vi "SerialPort.Manager.vi"(11 "Module Config":T4={"Name"="Serial Port", "Parent Q"=refnum, "Is Child?"=FALSE, "Index"=0, "Dirs"={"Root"=path "", "Config"=path "C:/ATE/Config", "Logs"=path "C:/ATE/Logs", "Reports"=path "C:/ATE/Reports", "App Data"=path "C:/ProgramData/MAIN"}, "Simulate"=FALSE, "SimCtrl"=refnum}) -> ()   [LabVIEW 2018]
uses:
  <vilib>/KATE/Module/Module Config.ctl
  <vilib>/KATE/Queues/Q.Element.ctl
  <vilib>/KATE/Module/Module.Working Dirs.ctl
  Controls/SerialPort.Status Enum.ctl
  Controls/SeroalPort.Config Settings.ctl
  <vilib>/KATE/Event Log/Event Notification/Event Log.Log Level.ctl
  <vilib>/KATE/Module/Module.SW Version Info.ctl
  <vilib>/KATE/Module/Window/Window.Task, Action.ctl
  Class/SerialPort.lvclass
  Controls/SerialPort.Parent Task Names.ctl
  Utils/Functions/FunctMgr/FunctMgr.lvclass
  <vilib>/Utility/sysdir.llb/System Directory Type.ctl
  <vilib>/KATE/Event Log/Event Notification/Event Log.Notification Type.ctl
  <vilib>/Utility/config.llb/Read Key (String).vi
  <vilib>/KATE/Config/Stored Controls/Class.SaveCtrls.lvclass
  <vilib>/KATE/Queues/Queue Utils.lvlib
  <vilib>/KATE/Module/Module Utils.lvlib
  <vilib>/KATE/Event Log/Event Log.lvlib
  <vilib>/KATE/Scheduler/Scheduler.lvlib
  <vilib>/KATE/Menu/Menu Utils.lvlib
  <vilib>/KATE/Config/Config Utils.lvlib
  <vilib>/KATE/Status/Status Utils.lvlib
  <vilib>/KATE/Files/File Utils.lvlib
  <vilib>/KATE/SeqMgr/SeqMgr.lvlib
  <vilib>/KATE/Event Log/Event Notification/Event Notification.lvclass
  <vilib>/Utility/config.llb/NI_LVConfig.lvlib
panel:
  in  "Main Tab":enum32{"Operate", "Maint"}(tab)
  in  "Data Tab":enum32{"Read/Write", "Config"}(tab)
  in  "Send Tab":bool
  in  "Save Log":bool
  out "Error Status":string
  in  "Clear Log":bool
  in  "Write":string
  out "Log":string
  in  "Log Size (Chars)":i32=100000
  in  "Auto Scroll":bool=TRUE
  out "Simulate Indication":string="Simulating Instruments"
  out "Q Dur ms":u32=100 caption="Dur(ms)"
  in  "Q Timeout ms":u32=5000 caption="Timeout ms"
  in  "Query":bool
  out "Q Data":string
  in  "Q Cmd":string="id" caption="Cmd"
  in  "Q MsgEnd":string="lhtx>" caption="MsgEnd"
  in  "VID":string="28DE"
  in  "PID":string
  in  "TermChar":string="\n\r" caption="Command Term Char"
  in  "Timeout ms (3sec)":u32=3000
  in  "Config":T1={"Baud Rate (115200)"=115200, "Data Bits (8)"=8, "Parity (0:none)"=enum."None", "Stop Bits (10: 1 bit)"=10, "Flow Control (0:none)"=enum."None", "Enable Term Char (T)"=TRUE, "Term Char(0xA = '\\n' = LF) "=10} {"Term Char(0xA = '\\n' = LF)" format="%.0x"; "Stop Bits (10: 1 bit)" items=["1.0"=10, "1.5"=15, "2.0"=20]; "Data Bits (8)" min=5 max=8 step=1}
  out "Status":string
  out "Error":errorcluster
  in  "Auto Find Port":bool=TRUE caption="Auto"
  in  "Logging Level":T2
  out "Rev":string="v1.0.0"
  in  "COM Port":refnum<visa-resource-name>
  in  "Disconnect":bool
  in  "Connect":bool
  out "State":T3
  in  "Leave Maint":bool
  # "Serial Port Manager"
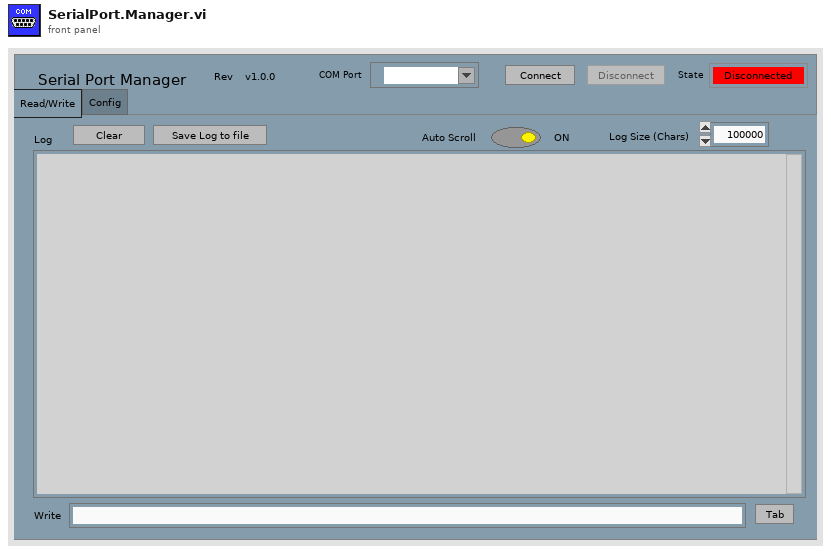
[diagram p1: front panel]
types:
  T1 = typedef "SeroalPort.Config Settings.ctl" = cluster{"Baud Rate (115200)":u32, "Data Bits (8)":u16, "Parity (0:none)":enum16{"None", "Odd", "Even", "Mark", "Space"}, "Stop Bits (10: 1 bit)":u16, "Flow Control (0:none)":enum16{"None", "XON/XOFF", "RTS/CTS", "XON/XOFF & RTS/CTS", "DTR/DSR", "XON/XOFF & DTR/DSR"}, "Enable Term Char (T)":bool, "Term Char(0xA = '\\n' = LF) ":u8}
  T2 = typedef "KATE_Lib.lvlib/Event Log.lvlib/Event Log.Log Level.ctl" = enum16{"Normal", "Verbose", "Debug0", "Debug1", "Debug2"}
  T3 = typedef "SerialPort.Status Enum.ctl" = enum16{"Disconnected", "Connecting", "Connected"}
  T4 = typedef "KATE_Lib.lvlib/Module Utils.lvlib/Module Config.ctl" = cluster{"Name":string, "Parent Q":refnum<queue>, "Is Child?":bool, "Index":i32, "Dirs":T5, "Simulate":bool, "SimCtrl":refnum<vi>}
  T5 = typedef "KATE_Lib.lvlib/Module Utils.lvlib/Module.Working Dirs.ctl" = cluster{"Root":path, "Config":path, "Logs":path, "Reports":path, "App Data":path}
  T6 = typedef "KATE_Lib.lvlib/Module Utils.lvlib/Module.SW Version Info.ctl" = cluster{"AppName":string, "Company":string, "Version":string, "Description":string, "PN":string}
  T7 = typedef "KATE_Lib.lvlib/Module Utils.lvlib/Module Sys Info.ctl" = cluster{"Main Q":refnum<queue>, "Exe":bool, "SW Rev":T6, "Self Ref":refnum<vi>, "Main Tab":refnum<vi>, "Pane":refnum<vi>, "Stop":cluster{"Ref":refnum<event-registration>, "Event":refnum<user-event>}, "Cfg":T4, "Services":cluster{"Name":string, "vi ref":refnum<vi>}[], "Menu Ref":refnum<k9>, "CtrlStates":refnum<class "Class.SaveCtrls.lvclass">, "Docs":cluster{"Tags":string[], "Paths":path[]}, "Log":refnum<class "Event Notification.lvclass">, "Test Controls":refnum<vi>[], "Child Modules":cluster{"Name":string, "vi ref":refnum<vi>}[], "SW Items":string[][], "AppData":refnum<class "Class.AppData.lvclass">, "Subscriptions":refnum<class "Subscription.lvclass">}
  T8 = typedef "SerialPort.Parent Task Names.ctl" = cluster{"Rcv":string, "Event":string}
  T9 = enum8{"Enabled", "Disabled", "Disabled and Grayed Out"}
  T10 = enum16{"open", "replace", "create", "open or create", "replace or create", "replace or create with confirmation"}
  T11 = cluster{"Port Name":string, "Config":T1, "Port Timeout ms (3000)":u32}
  T12 = typedef "KATE_Lib.lvlib/Event Log.lvlib/Event Log.Notification Type.ctl" = enum16{"Normal", "Warning", "Error", "Success"}
  T13 = cluster{"Child Modules":cluster{"VI Ref":refnum<vi>, "Name":string}[]}
  T14 = cluster{"Local Error":errorcluster, "Lnch":bool, "TBD":string, "App":cluster{"Child Modules":cluster{"VI Ref":refnum<vi>, "Name":string}[]}, "SerialPort":refnum<class "SerialPort.lvclass">, "Log":string, "Parent Tasks":T8, "FunctMgr":refnum<class "FunctMgr.lvclass">, "Ctrl Lock":bool}
  T15 = typedef "NI_LVConfig.lvlib/Config Data RefNum.ctl" = refnum<k1>
  T16 = typedef "System Directory Type.ctl" = i32
  T17 = typedef "KATE_Lib.lvlib/Module Utils.lvlib/Window.Task, Action.ctl" = enum16{"Resize()", "Show Panel(Bool)", "Show Scroll Bars(Bool)", "Dock to SubPanel(SubPanel Ref)", "Undock from SubPanel()", "Return to SubPanel()", "Go To Maint Tab()", "Show Maint Tab(Bool)", "Open Block Diagram()"}
  T18 = typedef "eventvkey.ctl" = enum16{"ASCII", "Enter", "Return", "Shift", "Ctrl", "Alt", "Cmd", "Opt", "Caps", "NumLock", "Clear", "Break", "Up", "Down", "Left", "Right", "Insert", "Delete", "Home", "End", "PageUp", "PageDown", "Escape", "Help", "Pause", "ScrollLock", "F1", "F2", "F3", "F4", "F5", "F6", "F7", "F8", "F9", "F10", "F11", "F12", "F13", "F14", "F15", "F16", "F17", "F18", "F19", "F20", "F21", "F22", "F23", "F24", "Play", "VolumeUp", "VolumeDown", "Mute", "Two Byte Char"}
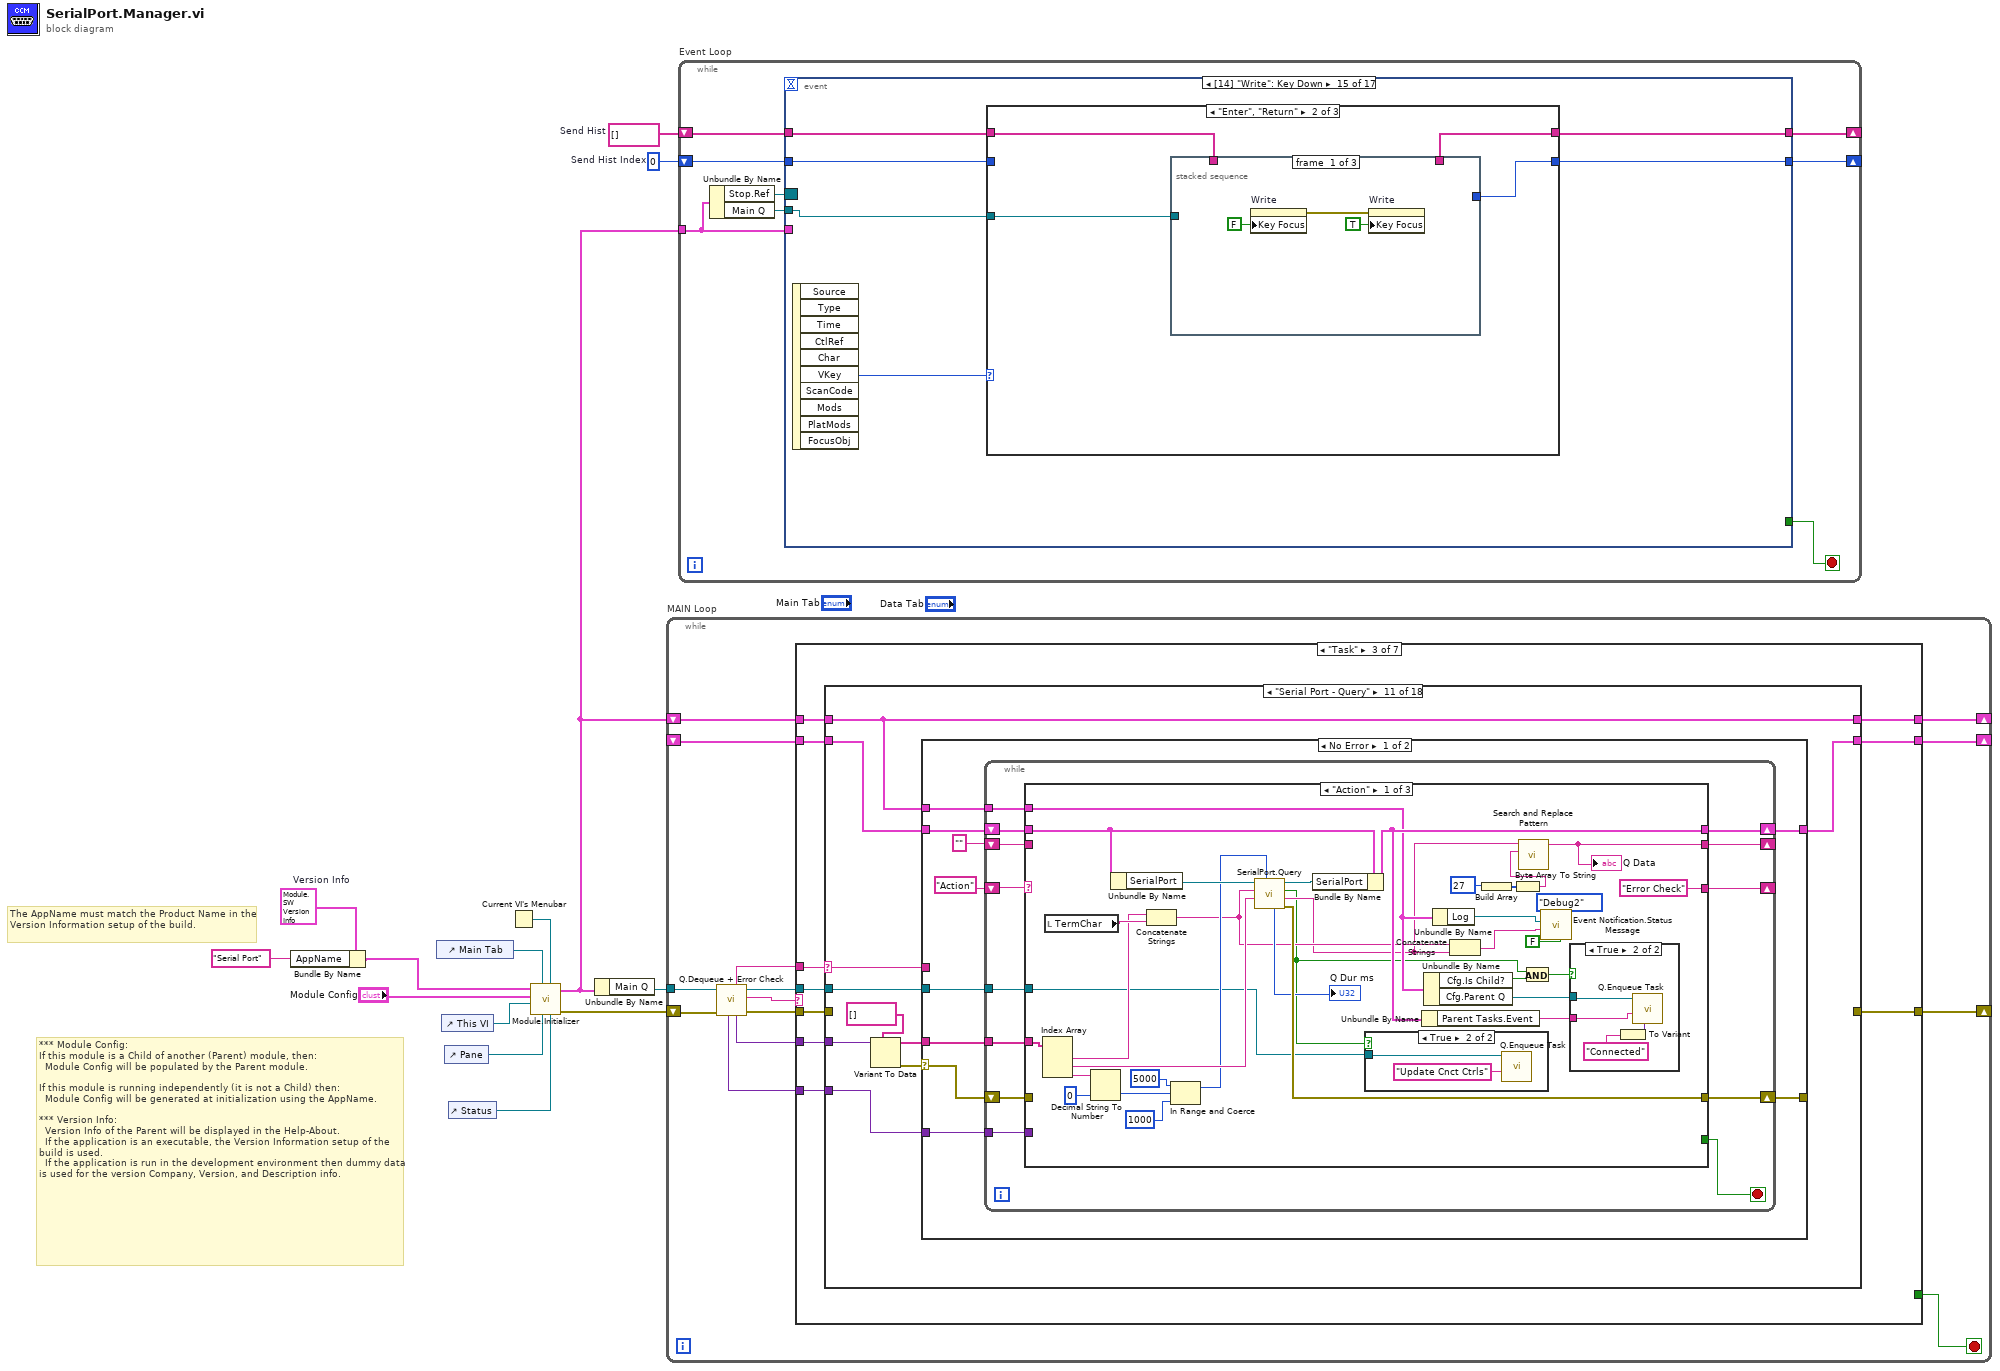
[diagram p0: block diagram]
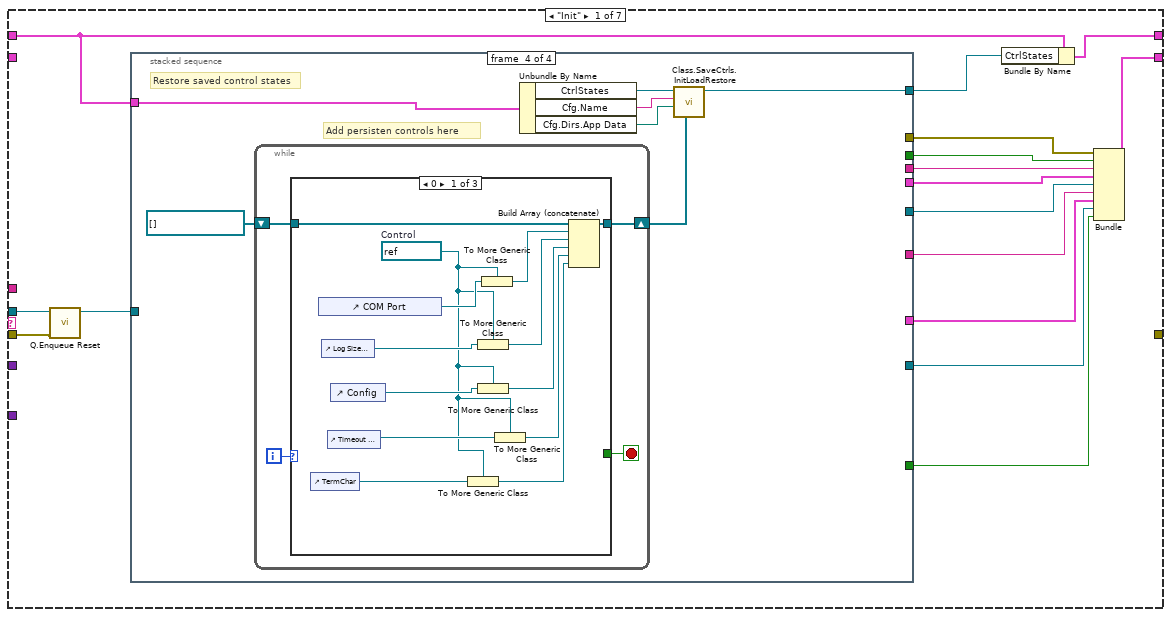
[diagram p2: hidden frame]
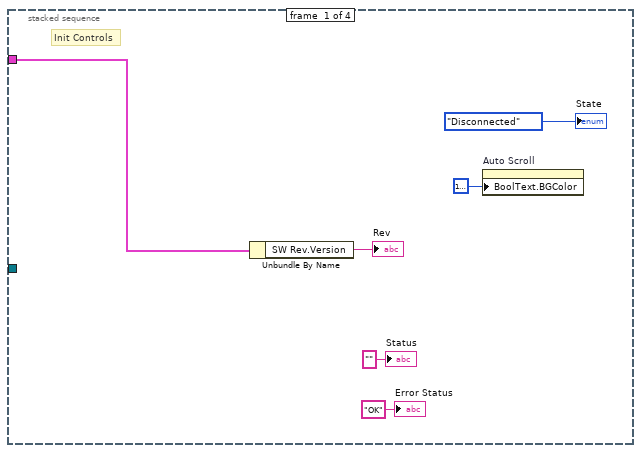
[diagram p3: hidden frame]
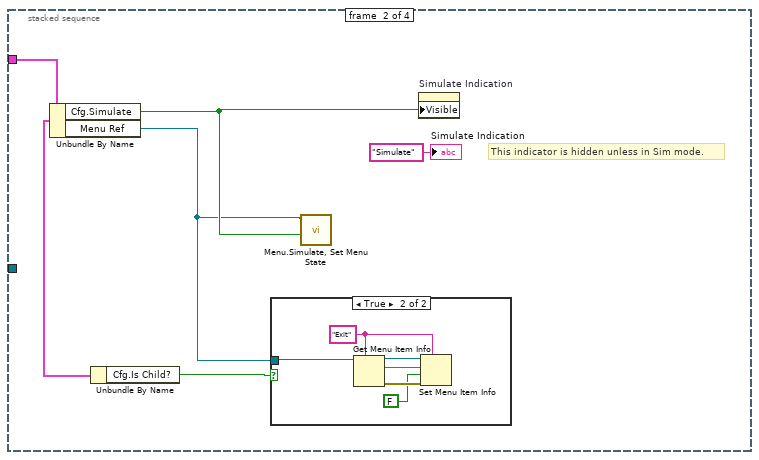
[diagram p4: hidden frame]
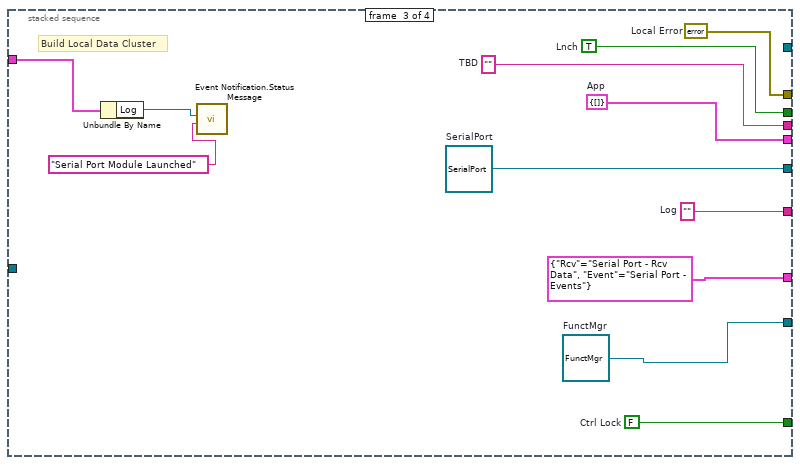
[diagram p6: hidden frame]
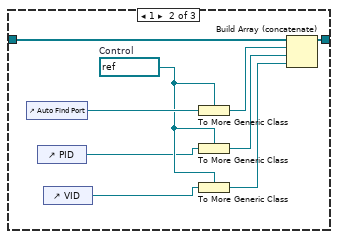
[diagram p7: hidden frame]
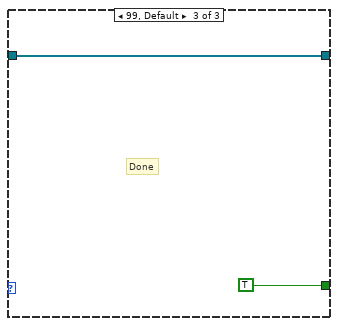
[diagram p8: hidden frame]
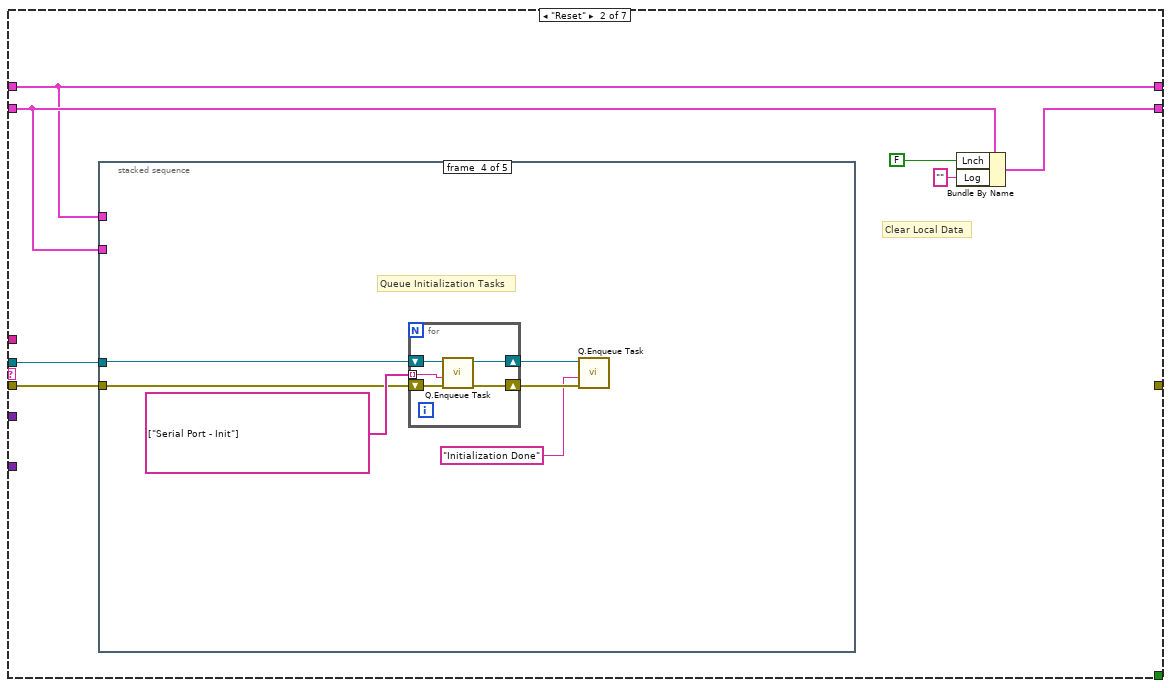
[diagram p9: hidden frame]
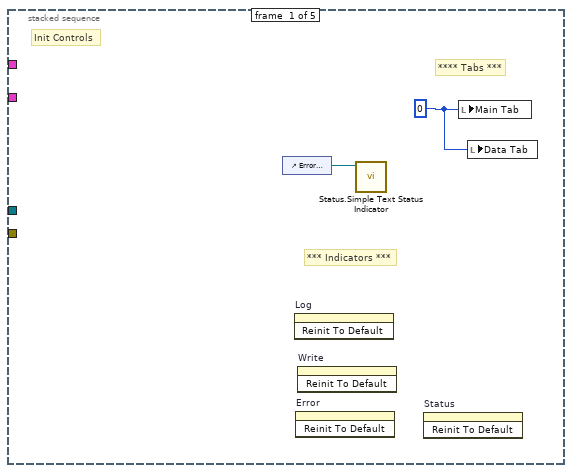
[diagram p10: hidden frame]
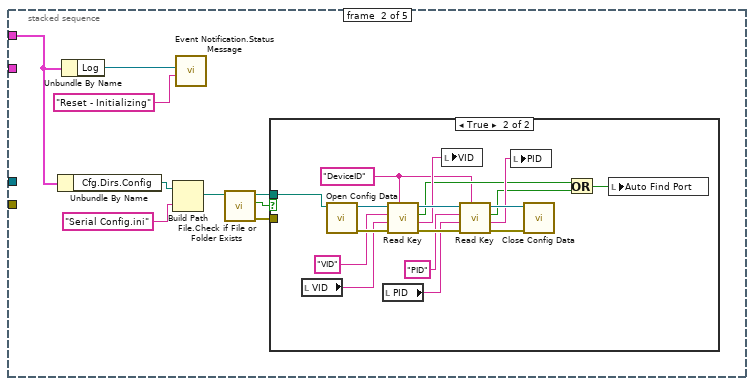
[diagram p11: hidden frame]
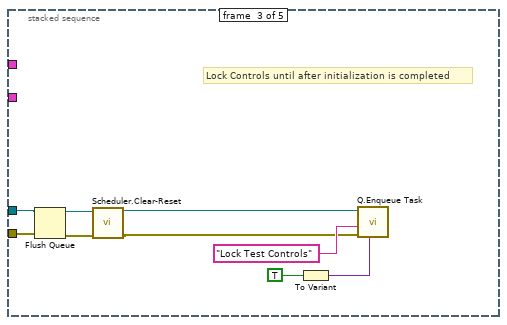
[diagram p13: hidden frame]
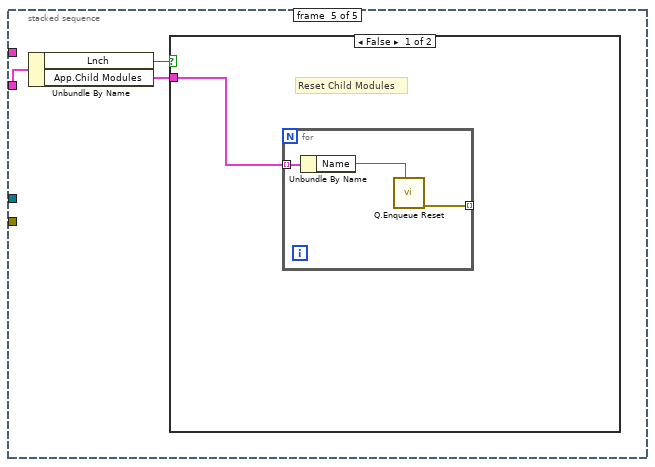
[diagram p14: hidden frame]
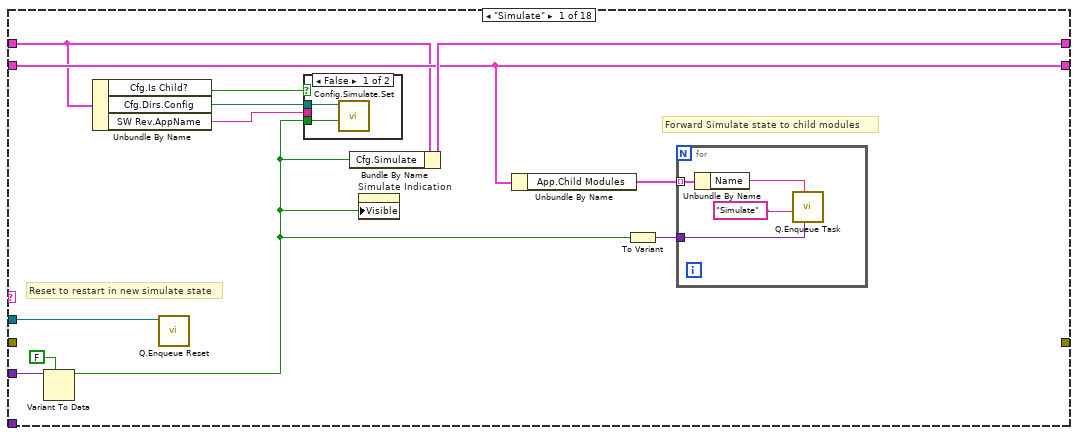
[diagram p16: hidden frame]
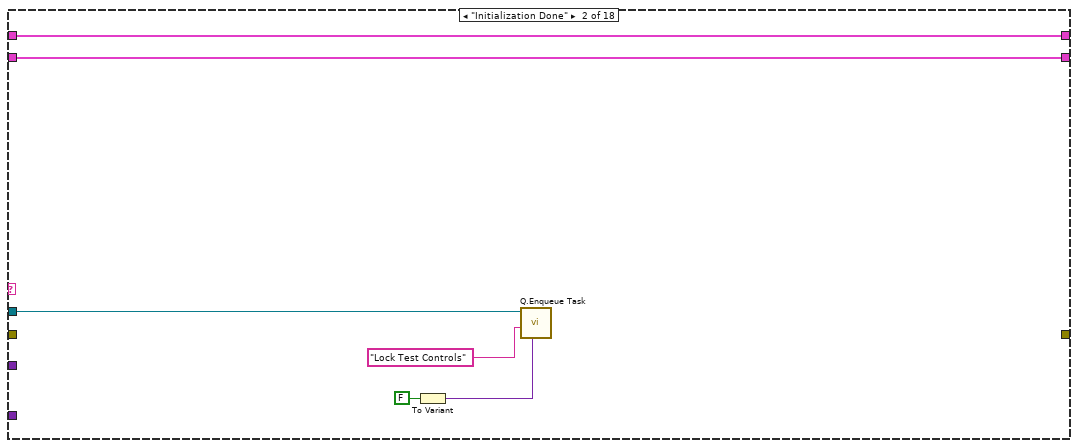
[diagram p18: hidden frame]
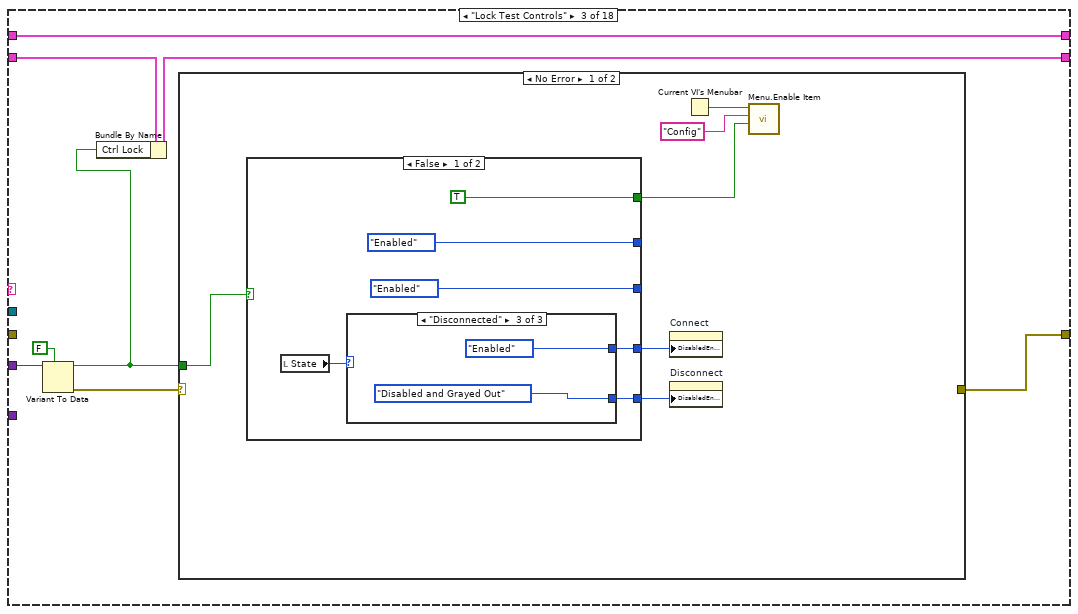
[diagram p19: hidden frame]
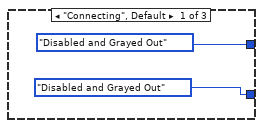
[diagram p20: hidden frame]
diagram:
  w2 = T6 {"AppName"="ModuleX", "Company"="CompanyX", "Version"="1.0", "Description"="This app is being developed.", "PN"=""}  # Version Info
  w5 = string[] []  # Send Hist
  w6 = 0  # Send Hist Index
  # "*** Module Config:\nIf this module is a Child of another (Parent) module, then:\n  Module Config will be populated by the Parent module.\n\nIf this module is running independently (it is not a Child) then:\n  Module Config will be generated at initialization using the AppName.\n\n*** Version Info:\n  Version Info of the Parent will be displayed in the Help-About.\n  If the application is an executable, the Version Information setup of the build is used.\n  If the application is run in the development environment then dummy data is used for the version Company, Version, and Description info."
  # "The AppName must match the Product Name in the Version Information setup of the build."
  n1 = Bundle By Name(cluster=w2, "AppName"="Serial Port") -> (w1:T6)
  n2 = control-ref of="Main Tab"() -> (w12:refnum<vi>)
  n3 = control-ref of="This VI"() -> (w11:refnum<vi>)
  n4 = control-ref of="Pane"() -> (w10:refnum<vi>)
  n5 = control-ref of="Status"() -> (w4:refnum<vi>)
  n6 = Current VI's Menubar() -> (w8:refnum<k9>)
  n7 = call <vilib>:"Module.Initializer.vi"("StatusTxtBx"=w4, "Menu Ref"=w8, "Pane"=w10, "Main Tab"=w12, "Self Ref"=w11, "Module Config"="Module Config", "SW Rev"=w1) -> ("error out"=w14:errorcluster, "Sys"=w9:T7)  [unwired: 3 in]
  n8 = Unbundle By Name(w9) -> ("Main Q"=w13:refnum<queue>)
  n9 = while "MAIN Loop" {
    shift-right: [w25] -> _
    shift-left: w14 -> [w23]
    shift-right: [w26] -> _
    shift-left: _ -> [w15]
    shift-right: [w27] -> _
    shift-left: w9 -> [w28]
    tunnel: w13 -> [w22]
    stop <- w17 stop-if-true
    n10 = call <vilib>:"Q.Dequeue + Error Check.vi"("Error In"=w23, "Q In"=w22) -> ("error out"=w24:errorcluster, "Cmd"=w21:string, "Q Out"=w20:refnum<queue>, "Data1"=w19:variant, "Sub"=w16:string, "Data2"=w18:variant)  [unwired: 4 in]
    n11 = case shown="\"Task\"" w21 {
      selector: w21 -> [_ _ _ _ _ w1003 _]
      tunnel: w15 -> [_ w112 w179 w758 w977 w997 w1065]
      tunnel: w28 -> [w39 w109 w180 w759 w978 w998 w1066]
      tunnel: [w40 w109 w178 w757 w976 w998 w1066] -> w27
      tunnel: [w42 w115 w177 w756 w975 w996 w1065] -> w26
      tunnel: [_ _ w171 w751 _ w1004 w1068] -> w25
      tunnel: w24 -> [w43 w113 w173 w752 _ w1001 _]
      tunnel: w20 -> [w44 w114 w174 w753 w981 w999 _]
      tunnel: w19 -> [_ _ w175 w754 w980 w1002 _]
      tunnel: w18 -> [_ _ w172 w750 w979 _ _]
      tunnel: w16 -> [_ _ w176 w755 w982 w1000 _]
      tunnel: [_ _ _ _ _ _ TRUE] -> w17
      frame "Init" {
        n12 = call <vilib>:"Q.Enqueue Reset.vi"("Error In"=w43, "Q In"=w44) -> ("Q Out"=w37:refnum<queue>)  [unwired: 8 in, 1 out]
        n13 = stacked-sequence {
          tunnel: [_ _ w65 _] -> w41
          tunnel: w39 -> [w49 w52 w64 w75]
          tunnel: [_ _ _ w74] -> w38
          tunnel: w37 -> [_ _ _ _]
          tunnel: [_ _ w73 _] -> w36
          tunnel: [_ _ w72 _] -> w35
          tunnel: [_ _ w71 _] -> w34
          tunnel: [_ _ w70 _] -> w33
          tunnel: [_ _ T8 {"Rcv"="Serial Port - Rcv Data", "Event"="Serial Port - Events"} ("Parent Tasks") _] -> w32
          tunnel: [_ _ w67 _] -> w31
          tunnel: [_ _ w68 _] -> w30
          tunnel: [_ _ w66 _] -> w29
          frame #0 {
            # "Init Controls"
            n14 = Unbundle By Name(w49) -> ("SW Rev.Version"=→"Rev":string)
            n15 = property on="Auto Scroll" class="Bool (strict)"("BoolText.BGColor"=u32 16777216 ("Boolean Text.Text Colors:Text Color")) -> ()  [unwired: 2 in, 2 out]
            "Status" <- "" ("Status")
            "Error Status" <- "OK" ("Error Status")
            "State" <- SerialPort.Status_Enum."Disconnected" ("State")
          }
          frame #1 {
            # "This indicator is hidden unless in Sim mode."
            n16 = Unbundle By Name(w52) -> ("Cfg.Simulate"=w54:bool, "Menu Ref"=w51:refnum<k9>)
            n17 = Unbundle By Name(w52) -> ("Cfg.Is Child?"=w53:bool)
            n18 = case shown="True" w53 {
              tunnel: w51 -> [_ w57]
              frame False {
              }
              frame True {
                w59 = "Exit"
                n19 = Get Menu Item Info(7:w59, 11:w57) -> (0:w58:errorcluster, 2:w60:string, 3:w61:refnum<k9>)  [unwired: 1 in, 4 out]
                n20 = Set Menu Item Info(7:w59, 8:w58, 9:FALSE ("enabled"), 10:w60, 11:w61) -> ()  [unwired: 2 in, 2 out]
              }
            }
            n21 = call <vilib>:"Menu.Simulate, Set Menu State.vi"("Sim Enable"=w54, "Menu Ref"=w51) -> ()  [unwired: 8 in, 2 out]
            n22 = property on="Simulate Indication" class="Str"("Visible"=w54) -> ()  [unwired: 2 in, 2 out]
            "Simulate Indication" <- "Simulate" ("Simulate Indication")
          }
          frame #2 {
            w65 = ""  # TBD
            w66 = errorcluster {"status"=FALSE, "code"=0, "source"=""}  # Local Error
            w67 = refnum<class "FunctMgr.lvclass"> refnum  # FunctMgr
            w68 = FALSE  # Ctrl Lock
            w70 = ""  # Log
            w71 = refnum<class "SerialPort.lvclass"> refnum  # SerialPort
            w72 = T13 {"Child Modules"=[]}  # App
            w73 = TRUE  # Lnch
            # "Build Local Data Cluster"
            n23 = Unbundle By Name(w64) -> ("Log"=w63:refnum<class "Event Notification.lvclass">)
            n24 = call <vilib>:"Event Notification.Status Message.vi"("Message"="Serial Port Module Launched", "Event Notification in"=w63) -> ()  [unwired: 10 in]
          }
          frame #3 {
            # "Add persisten controls here"
            # "Restore saved control states"
            n25 = while {
              shift-right: [w82] -> w76
              shift-left: refnum<vi>[] [] -> [w83]
              i -> [w84]
              stop <- w81 stop-if-true
              n26 = case shown="0" w84 {
                tunnel: w83 -> [w96 w105 w108]
                tunnel: [w97 w106 w108] -> w82
                tunnel: [_ _ TRUE] -> w81
                frame 0 {
                  w87 = refnum<vi> refnum  # Control
                  n27 = control-ref of="TermChar"() -> (w86:refnum<vi>)
                  n28 = control-ref of="COM Port"() -> (w94:refnum<vi>)
                  n29 = control-ref of="Log Size (Chars)"() -> (w93:refnum<vi>)
                  n30 = control-ref of="Timeout ms (3sec)"() -> (w90:refnum<vi>)
                  n31 = control-ref of="Config"() -> (w91:refnum<vi>)
                  n32 = To More Generic Class(target class=w87, reference=w86) -> (generic class reference=w85:refnum<vi>)
                  n33 = To More Generic Class(target class=w87, reference=w93) -> (generic class reference=w92:refnum<vi>)
                  n34 = To More Generic Class(target class=w87, reference=w91) -> (generic class reference=w89:refnum<vi>)
                  n35 = To More Generic Class(target class=w87, reference=w94) -> (generic class reference=w95:refnum<vi>)
                  n36 = To More Generic Class(target class=w87, reference=w90) -> (generic class reference=w88:refnum<vi>)
                  n37 = Build Array (concatenate)(w96, w95, w92, w89, w88, w85) -> (w97:refnum<vi>[])
                }
                frame 1 {
                  w100 = refnum<vi> refnum  # Control
                  n38 = control-ref of="Auto Find Port"() -> (w101:refnum<vi>)
                  n39 = control-ref of="PID"() -> (w99:refnum<vi>)
                  n40 = control-ref of="VID"() -> (w98:refnum<vi>)
                  n41 = To More Generic Class(target class=w100, reference=w101) -> (generic class reference=w104:refnum<vi>)
                  n42 = To More Generic Class(target class=w100, reference=w99) -> (generic class reference=w103:refnum<vi>)
                  n43 = To More Generic Class(target class=w100, reference=w98) -> (generic class reference=w102:refnum<vi>)
                  n44 = Build Array (concatenate)(w105, w104, w103, w102) -> (w106:refnum<vi>[])
                }
                frame 99, Default {
                  # "Done"
                }
              }
            }
            n45 = Unbundle By Name(w75) -> ("CtrlStates"=w77:refnum<class "Class.SaveCtrls.lvclass">, "Cfg.Name"=w79:string, "Cfg.Dirs.App Data"=w78:path)
            n46 = call-dynamic "Class.SaveCtrls.InitLoadRestore.vi"("Ctrl Array"=w76, "Module Data Dir"=w78, "Module Name"=w79, "CtrlStates In"=w77) -> ("CtrlStates"=w74:refnum<class "Class.SaveCtrls.lvclass">)  [unwired: 6 in, 1 out]
          }
        }
        n47 = Bundle By Name(cluster=w39, "CtrlStates"=w38) -> (w40:T7)
        n48 = Bundle("Local Error"=w29, "Lnch"=w36, "TBD"=w41, "App"=w35, "SerialPort"=w34, "Log"=w33, "Parent Tasks"=w32, "FunctMgr"=w31, "Ctrl Lock"=w30) -> (w42:T14)  [unwired: 1 in]
      }
      frame "Reset" {
        # "Clear Local Data"
        n49 = stacked-sequence {
          tunnel: w114 -> [_ _ w145 w153 _]
          tunnel: w113 -> [_ _ w144 w157 _]
          tunnel: w112 -> [_ _ _ _ w166]
          tunnel: w109 -> [_ w124 _ _ _]
          frame #0 {
            w117 = 0
            # "*** Indicators ***"
            # "**** Tabs ***"
            # "Init Controls"
            n50 = control-ref of="Error Status"() -> (w116:refnum<vi>)
            n51 = invoke on="Log" class="Str" method="Reinit To Default"() -> ()  [unwired: 3 in, 3 out]
            n52 = invoke on="Error" class="Clust (strict)" method="Reinit To Default"() -> ()  [unwired: 3 in, 3 out]
            n53 = invoke on="Write" class="Str" method="Reinit To Default"() -> ()  [unwired: 3 in, 3 out]
            n54 = call <vilib>:"Status.Simple Text Status Indicator.vi"("Status TextBox"=w116) -> ()  [unwired: 10 in, 1 out]
            n55 = invoke on="Status" class="Str" method="Reinit To Default"() -> ()  [unwired: 3 in, 3 out]
            n56 = local write "Main Tab"(w117) -> ()
            n57 = local write "Data Tab"(w117) -> ()
          }
          frame #1 {
            n58 = Unbundle By Name(w124) -> ("Cfg.Dirs.Config"=w118:path)
            n59 = Unbundle By Name(w124) -> ("Log"=w126:refnum<class "Event Notification.lvclass">)
            n60 = Build Path(base path=w118, name or relative path="Serial Config.ini" ("Message")) -> (appended path=w120:path)
            n61 = call <vilib>:"Event Notification.Status Message.vi"("Message"="Reset - Initializing", "Event Notification in"=w126) -> ()  [unwired: 10 in]
            n62 = call <vilib>:"File.Check if File or Folder Exists.vi"("Path"=w120) -> ("error out"=w121:errorcluster, "Exists"=w123:bool, "Dup Path"=w122:path)  [unwired: 6 in, 2 out]
            n63 = case shown="True" w123 {
              tunnel: w122 -> [_ w131]
              tunnel: w121 -> [_ _]
              frame False {
              }
              frame True {
                w127 = "DeviceID"
                n64 = local read "VID"() -> (w136:string)
                n65 = call <vilib>:"Open Config Data.vi"("configuration file path"=w131) -> ("error out"=w143:errorcluster, "refnum"=w142:T15)  [unwired: 8 in, 1 out]
                n66 = local read "PID"() -> (w134:string)
                n67 = call-poly <vilib>:"Read Key.vi"("section"=w127, "error in (no error)"=w143, "default value"=w136, "key"="VID", "refnum"=w142) -> ("error out"=w139:errorcluster, "value"=w132:string, "found?"=w130:bool, "refnum out"=w140:T15)  [unwired: 3 in]
                n68 = local write "VID"(w132) -> ()
                n69 = call-poly <vilib>:"Read Key.vi"("section"=w127, "error in (no error)"=w139, "default value"=w134, "key"="PID", "refnum"=w140) -> ("error out"=w138:errorcluster, "value"=w133:string, "found?"=w129:bool, "refnum out"=w141:T15)  [unwired: 3 in]
                n70 = local write "PID"(w133) -> ()
                n71 = call <vilib>:"Close Config Data.vi"("error in (no error)"=w138, "refnum"=w141) -> ()  [unwired: 8 in, 2 out]
                n72 = Or(x=w130, y=w129) -> (x .or. y?=w128:bool)
                n73 = local write "Auto Find Port"(w128) -> ()
              }
            }
          }
          frame #2 {
            # "Lock Controls until after initialization is completed"
            n74 = Flush Queue(queue=w145, error in (no error)=w144) -> (queue out=w146:refnum<queue>, error out=w149:errorcluster)  [unwired: 1 out]
            n75 = call <vilib>:"Scheduler.Clear-Reset.vi"("error in"=w149, "Q In"=w146) -> ("error out"=w147:errorcluster, "Q Out"=w148:refnum<queue>)  [unwired: 8 in]
            n76 = To Variant(anything=TRUE) -> (Variant=w151:variant)
            n77 = call <vilib>:"Q.Enqueue Task.vi"("Data1"=w151, "Error In"=w147, "Task Name"="Lock Test Controls", "Q In"=w148) -> ()  [unwired: 6 in, 2 out]
          }
          frame #3 {
            # "Queue Initialization Tasks"
            n78 = for {
              shift-right: [w161] -> w155
              shift-left: w157 -> [w162]
              tunnel: string[] ["Serial Port - Init"] -> [w159] mode=indexing
              shift-right: [w160] -> w156
              shift-left: w153 -> [w163]
              n79 = call <vilib>:"Q.Enqueue Task.vi"("Error In"=w162, "Task Name"=w159, "Q In"=w163) -> ("error out"=w161:errorcluster, "Q Out"=w160:refnum<queue>)  [unwired: 7 in]
            }
            n80 = call <vilib>:"Q.Enqueue Task.vi"("Error In"=w155, "Task Name"="Initialization Done", "Q In"=w156) -> ()  [unwired: 7 in, 2 out]
          }
          frame #4 {
            n81 = Unbundle By Name(w166) -> ("Lnch"=w165:bool, "App.Child Modules"=w164:cluster{"VI Ref":refnum<vi>, "Name":string}[])
            n82 = case shown="False" w165 {
              tunnel: w164 -> [w167 _]
              frame False {
                # "Reset Child Modules"
                n83 = for {
                  tunnel: w167 -> [w170] mode=indexing
                  tunnel: [w168] -> _ mode=indexing
                  n84 = Unbundle By Name(w170) -> ("Name"=w169:string)
                  n85 = call <vilib>:"Q.Enqueue Reset.vi"("Q Name"=w169) -> ("error out"=w168:errorcluster)  [unwired: 9 in, 1 out]
                }
              }
              frame True {
                # "Do not reset at launch.\nThey are already reset"
              }
            }
          }
        }
        n86 = Bundle By Name(cluster=w112, "Lnch"=FALSE ("Test.Running"), "Log"="") -> (w115:T14)
      }
      frame "Task" {
        n87 = case shown="\"Serial Port - Query\"" w176 {
          selector: w176 -> [_ _ _ _ _ _ _ _ _ _ w433 w548 _ _ _ _ _ w744]
          tunnel: w180 -> [w185 w204 w212 w248 w255 w267 w276 w277 w377 w392 w437 w544 w647 w679 w706 w717 w730 w745]
          tunnel: w179 -> [w189 w199 w207 w242 w254 w266 w271 w283 w374 w399 w436 w549 w648 w667 w705 w713 w729 w746]
          tunnel: [w190 w204 w212 w248 w255 w267 w276 w277 w377 w392 w437 w544 w647 w679 w706 w717 w730 w745] -> w178
          tunnel: [w189 w199 w206 w241 w254 w265 w272 w282 w374 w393 w435 w550 w652 w666 w705 w712 w729 w746] -> w177
          tunnel: w175 -> [w192 _ w211 _ w253 _ _ _ _ _ w431 w553 _ w677 _ w709 w731 w743]
          tunnel: w174 -> [w186 w203 _ w239 w251 w264 _ w284 _ w397 w434 w547 w659 _ _ _ _ _]
          tunnel: w173 -> [_ _ _ _ _ _ _ w278 _ _ _ _ _ _ _ _ _ w741]
          tunnel: w172 -> [_ _ _ _ _ _ _ w280 _ _ w428 w545 _ _ _ w710 _ w742]
          tunnel: [_ _ w208 w240 _ w260 w273 w281 _ w398 _ w551 _ _ _ w711 w728 w740] -> w171
          frame "Simulate" {
            # "Reset to restart in new simulate state"
            # "Forward Simulate state to child modules"
            n88 = Variant To Data(type=FALSE, Variant=w192) -> (data=w182:bool)  [unwired: 1 in, 1 out]
            n89 = Unbundle By Name(w185) -> ("Cfg.Is Child?"=w181:bool, "Cfg.Dirs.Config"=w184:path, "SW Rev.AppName"=w183:string)
            n90 = call <vilib>:"Q.Enqueue Reset.vi"("Q In"=w186) -> ()  [unwired: 9 in, 2 out]
            n91 = case shown="False" w181 {
              tunnel: w184 -> [w194 _]
              tunnel: w183 -> [_ _]
              tunnel: w182 -> [w193 _]
              frame False {
                n92 = call <vilib>:"Config.Simulate.Set.vi"("Simulate"=w193, "Config Folder"=w194) -> ()  [unwired: 9 in, 1 out]
              }
              frame True {
              }
            }
            n93 = Bundle By Name(cluster=w185, "Cfg.Simulate"=w182) -> (w190:T7)
            n94 = property on="Simulate Indication" class="Str"("Visible"=w182) -> ()  [unwired: 2 in, 2 out]
            n95 = Unbundle By Name(w189) -> ("App.Child Modules"=w188:cluster{"VI Ref":refnum<vi>, "Name":string}[])
            n96 = To Variant(anything=w182) -> (Variant=w187:variant)
            n97 = for {
              tunnel: w188 -> [w198] mode=indexing
              tunnel: w187 -> [w195]
              n98 = Unbundle By Name(w198) -> ("Name"=w197:string)
              n99 = call <vilib>:"Q.Enqueue Task.vi"("Data1"=w195, "Q Name"=w197, "Task Name"="Simulate") -> ()  [unwired: 7 in, 2 out]
            }
          }
          frame "Initialization Done" {
            n100 = To Variant(anything=FALSE) -> (Variant=w201:variant)
            n101 = call <vilib>:"Q.Enqueue Task.vi"("Data1"=w201, "Task Name"="Lock Test Controls", "Q In"=w203) -> ()  [unwired: 7 in, 2 out]
          }
          frame "Lock Test Controls" {
            n102 = Variant To Data(type=FALSE, Variant=w211) -> (data=w205:bool, error out=w209:errorcluster)  [unwired: 1 in]
            n103 = Bundle By Name(cluster=w207, "Ctrl Lock"=w205) -> (w206:T14)
            n104 = case shown="No Error" w209 {
              selector: w209 -> [_ w235]
              tunnel: w205 -> [w218 _]
              tunnel: [_ w235] -> w208
              frame No Error {
                n105 = case shown="False" w218 {
                  tunnel: [T9."Enabled" ("Disabled") T9."Disabled and Grayed Out" ("Disabled")] -> _
                  tunnel: [T9."Enabled" ("Disabled") T9."Disabled" ("Disabled")] -> _
                  tunnel: [TRUE ("Enable") FALSE ("Enable")] -> w215
                  tunnel: [w221 w231] -> w214
                  tunnel: [w220 w231] -> w213
                  frame False {
                    n106 = local read "State"() -> (w219:T3)
                    n107 = case shown="\"Disconnected\"" w219 {
                      tunnel: [T9."Disabled and Grayed Out" ("Disabled") T9."Disabled and Grayed Out" ("Disabled") T9."Enabled" ("Disabled")] -> w221
                      tunnel: [T9."Disabled and Grayed Out" ("Disabled") T9."Enabled" ("Disabled") T9."Disabled and Grayed Out" ("Disabled")] -> w220
                      frame "Connecting", Default {
                      }
                      frame "Connected" {
                      }
                      frame "Disconnected" {
                      }
                    }
                  }
                  frame True {
                    w231 = T9."Disabled and Grayed Out" ("Disabled")
                  }
                }
                n108 = property on="Connect" class="Bool"("DisabledEnum"=w214) -> ()  [unwired: 2 in, 2 out]
                n109 = property on="Disconnect" class="Bool"("DisabledEnum"=w213) -> ()  [unwired: 2 in, 2 out]
                n110 = Current VI's Menubar() -> (w216:refnum<k9>)
                n111 = call <vilib>:"Menu.Enable Item.vi"("Enable"=w215, "Tag"="Config", "Menu Ref"=w216) -> ()  [unwired: 7 in, 2 out]
              }
              frame Error {
              }
            }
          }
          frame "Serial Port - Init" {
            n112 = call <vilib>:"Scheduler.Delete Task.vi"("Sched Name"="Serial Port - Read", "Q In"=w239) -> ("Q Out"=w236:refnum<queue>)  [unwired: 8 in, 1 out]
            n113 = call <vilib>:"Q.Enqueue Task.vi"("Task Name"="Update Cnct Ctrls", "Q In"=w236) -> ()  [unwired: 8 in, 2 out]
            n114 = Unbundle By Name(w242) -> ("SerialPort"=w246:refnum<class "SerialPort.lvclass">)
            n115 = control-ref of="State"() -> (w247:refnum<vi>)
            n116 = call "SerialPort.Config_All.vi"("State Ctrl Ref"=w247, "Config"="Config", "Com Port"="COM Port", "SerialPort in"=w246) -> ("error out"=w240:errorcluster, "SerialPort out"=w243:refnum<class "SerialPort.lvclass">)  [unwired: 6 in]
            n117 = Bundle By Name(cluster=w242, "SerialPort"=w243) -> (w241:T14)
          }
          frame "Serial Port - Set Config" {
            n118 = Variant To Data(type=T1 {"Baud Rate (115200)"=115200, "Data Bits (8)"=8, "Parity (0:none)"=enum."None", "Stop Bits (10: 1 bit)"=10, "Flow Control (0:none)"=enum."None", "Enable Term Char (T)"=TRUE, "Term Char(0xA = '\\n' = LF) "=10} ("Config"), Variant=w253) -> (data=w250:T1, error out=w249:errorcluster)  [unwired: 1 in]
            n119 = case shown="No Error" w249 {
              tunnel: w251 -> [w257 _]
              tunnel: w250 -> [w256 _]
              frame No Error {
                n120 = local write "Config"(w256) -> ()
                n121 = call <vilib>:"Q.Enqueue Task.vi"("Task Name"="Serial Port - Init" ("Name"), "Q In"=w257) -> ()  [unwired: 8 in, 2 out]
              }
              frame Error {
              }
            }
          }
          frame "Serial Port - Set Timeout" {
            n122 = call <vilib>:"Scheduler.Delete Task.vi"("Sched Name"="Serial Port - Read", "Q In"=w264) -> ()  [unwired: 8 in, 2 out]
            n123 = Unbundle By Name(w266) -> ("SerialPort"=w262:refnum<class "SerialPort.lvclass">)
            n124 = call "SerialPort.Config_Timeout.vi"("Timeout ms (3sec)"="Timeout ms (3sec)", "SerialPort in"=w262) -> ("error out"=w260:errorcluster, "SerialPort out"=w261:refnum<class "SerialPort.lvclass">)  [unwired: 8 in]
            n125 = Bundle By Name(cluster=w266, "SerialPort"=w261) -> (w265:T14)
          }
          frame "Serial Port - Auto Find" {
            n126 = Unbundle By Name(w271) -> ("SerialPort"=w275:refnum<class "SerialPort.lvclass">)
            n127 = call "SerialPort.Auto Find Port.vi"("PID"="PID", "VID"="VID", "SerialPort in"=w275) -> ("error out"=w273:errorcluster, "VISA resource name"=w270:refnum<visa-resource-name>, "SerialPort out"=w274:refnum<class "SerialPort.lvclass">)  [unwired: 6 in]
            n128 = Bundle By Name(cluster=w271, "SerialPort"=w274) -> (w272:T14)
            n129 = local write "COM Port"(w270) -> ()
          }
          frame "Serial Port - Connect" {
            n130 = while {
              shift-right: [w289] -> w282
              shift-left: w283 -> [w290]
              shift-right: [w291] -> w281
              shift-left: w278 -> [w292]
              shift-right: [w293] -> _
              shift-left: "Action" -> [w294]
              tunnel: w284 -> [w287]
              tunnel: w280 -> [w286]
              tunnel: w277 -> [w285]
              stop <- w288 stop-if-true
              n131 = case shown="\"Action\"" w294 {
                tunnel: ["Error Check" "Log Event" "Return" _] -> w293
                tunnel: w292 -> [_ w319 w341 w358]
                tunnel: [w303 w320 w341 w358] -> w291
                tunnel: w290 -> [w305 w318 w343 w360]
                tunnel: [w304 w318 w343 w359] -> w289
                tunnel: [_ _ _ TRUE] -> w288
                tunnel: w287 -> [w301 w321 _ _]
                tunnel: w286 -> [_ _ _ w361]
                tunnel: w285 -> [_ w317 w344 _]
                frame "Action" {
                  n132 = local read "Auto Find Port"() -> (w297:bool)
                  n133 = Unbundle By Name(w305) -> ("SerialPort"=w299:refnum<class "SerialPort.lvclass">)
                  n134 = local read "PID"() -> (w295:string)
                  n135 = local read "VID"() -> (w296:string)
                  n136 = call <vilib>:"Q.Enqueue Task.vi"("Task Name"="Update Cnct Ctrls" ("Name"), "Q In"=w301) -> ()  [unwired: 8 in, 2 out]
                  n137 = case shown="True" w297 {
                    tunnel: [w309 w315] -> w300
                    tunnel: w299 -> [w309 w314]
                    tunnel: [_ w313] -> w298
                    tunnel: w296 -> [_ w311]
                    tunnel: w295 -> [_ w310]
                    frame False {
                    }
                    frame True {
                      n138 = call "SerialPort.Auto Find Port.vi"("PID"=w310, "VID"=w311, "SerialPort in"=w314) -> ("error out"=w313:errorcluster, "VISA resource name"=w312:refnum<visa-resource-name>, "SerialPort out"=w315:refnum<class "SerialPort.lvclass">)  [unwired: 6 in]
                      n139 = local write "COM Port"(w312) -> ()
                    }
                  }
                  n140 = call "SerialPort.Connect.vi"("error in (no error)"=w298, "SerialPort in"=w300) -> ("error out"=w303:errorcluster, "SerialPort out"=w307:refnum<class "SerialPort.lvclass">)  [unwired: 7 in, 1 out]
                  n141 = Bundle By Name(cluster=w305, "Log"="", "SerialPort"=w307) -> (w304:T14)
                  n142 = invoke on="Log" class="Str" method="Reinit To Default"() -> ()  [unwired: 3 in, 3 out]
                }
                frame "Error Check" {
                  n143 = local read "COM Port"() -> (w316:refnum<visa-resource-name>)
                  n144 = case shown="Error" w319 {
                    selector: w319 -> [_ w340]
                    tunnel: [_ w340] -> w320
                    tunnel: w321 -> [w329 w339]
                    tunnel: w317 -> [w328 w333]
                    tunnel: w316 -> [w323 w332]
                    frame No Error {
                      w330 = "Serial Port - Read" ("Name")
                      n145 = Unbundle By Name(w328) -> ("Log"=w326:refnum<class "Event Notification.lvclass">)
                      n146 = Format Into String(format string="Connected to \"%s\".", w323) -> (resulting string=w325:string)  [unwired: 2 in, 1 out]
                      n147 = invoke on="Error" class="Clust (strict)" method="Reinit To Default"() -> ()  [unwired: 3 in, 3 out]
                      n148 = call <vilib>:"Event Notification.Status Message.vi"("Level"=Event_Log.Log_Level."Verbose", "Message"=w325, "Event Notification in"=w326) -> ()  [unwired: 9 in]
                      n149 = call <vilib>:"Scheduler.AddTask.vi"("Interval(s)"=0.1, "Task Name"=w330, "Sched Name"=w330, "Q In"=w329) -> ()  [unwired: 6 in, 2 out]
                    }
                    frame Error {
                      n150 = Unbundle By Name(w333) -> ("Log"=w335:refnum<class "Event Notification.lvclass">)
                      n151 = Format Into String(format string="Failed to connect to \"%s\".", w332) -> (resulting string=w334:string)  [unwired: 2 in, 1 out]
                      n152 = call <vilib>:"Scheduler.Delete Task.vi"("Sched Name"="Serial Port - Read" ("Name"), "Q In"=w339) -> ()  [unwired: 8 in, 2 out]
                      n153 = call <vilib>:"Event Notification.Status Message.vi"("Level"=Event_Log.Log_Level."Verbose", "Message"=w334, "Event Notification in"=w335) -> ()  [unwired: 9 in]
                    }
                  }
                }
                frame "Log Event" {
                  n154 = control-ref of="Error Status"() -> (w342:refnum<vi>)
                  n155 = Unbundle By Name(w343) -> ("Parent Tasks.Event"=w348:string)
                  n156 = Unbundle By Name(w344) -> ("Cfg.Is Child?"=w346:bool, "Cfg.Parent Q"=w347:refnum<queue>)
                  n157 = call <vilib>:"Status.Simple Text Status Indicator.vi"("error in"=w341, "Status TextBox"=w342) -> ()  [unwired: 9 in, 1 out]
                  n158 = case shown="True" w346 {
                    tunnel: w347 -> [_ w352]
                    tunnel: w348 -> [_ w351]
                    tunnel: w341 -> [_ w350]
                    frame False {
                    }
                    frame True {
                      n159 = case shown="No Error" w350 {
                        tunnel: ["Connected" ("Name") w356] -> w349
                        frame No Error {
                        }
                        frame Error {
                          n160 = local read "COM Port"() -> (w355:refnum<visa-resource-name>)
                          n161 = Format Into String(format string="Unsuccessful connection attempt on port \"%s\"." ("Name"), w355) -> (resulting string=w356:string)  [unwired: 2 in, 1 out]
                        }
                      }
                      n162 = To Variant(anything=w349) -> (Variant=w353:variant)
                      n163 = call <vilib>:"Q.Enqueue Task.vi"("Data1"=w353, "Task Name"=w351, "Q In"=w352) -> ()  [unwired: 7 in, 2 out]
                    }
                  }
                }
                frame "Return", Default {
                  n164 = Variant To Data(type="", Variant=w361) -> (data=w364:string, error out=w363:errorcluster)  [unwired: 1 in]
                  n165 = case shown="No Error" w363 {
                    tunnel: w360 -> [w369 w372]
                    tunnel: [w368 w372] -> w359
                    tunnel: w364 -> [w367 _]
                    tunnel: w358 -> [w366 _]
                    frame No Error {
                      n166 = Unbundle By Name(w369) -> ("FunctMgr"=w371:refnum<class "FunctMgr.lvclass">)
                      n167 = call "FunctMgr.Pop and Return.vi"("error in (no error)"=w366, "Ret ID"=w367, "FunctMgr in"=w371) -> ("FunctMgr out"=w370:refnum<class "FunctMgr.lvclass">)  [unwired: 6 in, 2 out]
                      n168 = Bundle By Name(cluster=w369, "FunctMgr"=w370) -> (w368:T14)
                    }
                    frame Error {
                      # "No return message ID so do nothing."
                    }
                  }
                }
              }
            }
          }
          frame "Update Cnct Ctrls" {
            n169 = Unbundle By Name(w374) -> ("Ctrl Lock"=w373:bool)
            n170 = case shown="False" w373 {
              tunnel: [w380 w387] -> w376
              tunnel: [w379 w387] -> w375
              frame False {
                n171 = local read "State"() -> (w378:T3)
                n172 = case shown="\"Disconnected\"" w378 {
                  tunnel: [T9."Disabled and Grayed Out" ("Disabled") T9."Disabled and Grayed Out" ("Disabled") T9."Enabled" ("Disabled")] -> w379
                  tunnel: [T9."Disabled and Grayed Out" ("Disabled") T9."Enabled" ("Disabled") T9."Disabled and Grayed Out" ("Disabled")] -> w380
                  frame "Connecting", Default {
                  }
                  frame "Connected" {
                  }
                  frame "Disconnected" {
                  }
                }
              }
              frame True {
                w387 = T9."Disabled and Grayed Out" ("Disabled")
              }
            }
            n173 = property on="Connect" class="Bool"("DisabledEnum"=w375) -> ()  [unwired: 2 in, 2 out]
            n174 = property on="Disconnect" class="Bool"("DisabledEnum"=w376) -> ()  [unwired: 2 in, 2 out]
          }
          frame "Serial Port - Read" {
            n175 = Unbundle By Name(w399) -> ("SerialPort"=w395:refnum<class "SerialPort.lvclass">)
            n176 = Unbundle By Name(w392) -> ("Log"=w391:refnum<class "Event Notification.lvclass">)
            n177 = call "SerialPort.Read.vi"("SerialPort in"=w395) -> ("error out"=w394:errorcluster, "Data"=w390:string, "SerialPort out"=w396:refnum<class "SerialPort.lvclass">)  [unwired: 7 in, 1 out]
            n178 = call <vilib>:"Event Notification.Status Message.vi"("Display"=FALSE, "Level"=Event_Log.Log_Level."Debug2", "Message"=w390, "Event Notification in"=w391) -> ()  [unwired: 8 in]
            n179 = Bundle By Name(cluster=w399, "SerialPort"=w396) -> (w393:T14)
            n180 = case shown="No Error" w394 {
              selector: w394 -> [_ w427]
              tunnel: [_ w427] -> w398
              tunnel: w397 -> [w405 w426]
              tunnel: w390 -> [w401 _]
              tunnel: w392 -> [w410 _]
              tunnel: w393 -> [w409 _]
              frame No Error {
                w406 = "Serial Port - Read" ("Name")
                n181 = Build Array(u8 27) -> (w404:u8[])
                n182 = Byte Array To String(unsigned byte array=w404) -> (string=w403:string)
                n183 = call <vilib>:"Search and Replace Pattern.vi"("string"=w401, "regular expression (\"\")"=w403) -> ("result string"=w400:string)  [unwired: 3 in, 1 out]
                n184 = Empty String/Path?(string/path=w400) -> (empty?=w408:bool)
                n185 = case shown="False" w408 {
                  tunnel: w400 -> [w418 _]
                  tunnel: w410 -> [w416 _]
                  tunnel: w409 -> [w413 _]
                  tunnel: w405 -> [w411 _]
                  frame False {
                    # "If is child, forward data"
                    n186 = To Variant(anything=w418) -> (Variant=w417:variant)
                    n187 = Unbundle By Name(w413) -> ("Parent Tasks.Rcv"=w412:string)
                    n188 = Unbundle By Name(w416) -> ("Cfg.Is Child?"=w415:bool, "Cfg.Parent Q"=w414:refnum<queue>)
                    n189 = call <vilib>:"Q.Enqueue Task.vi"("Data1"=w417, "Task Name"="Display Data" ("Name"), "Q In"=w411) -> ()  [unwired: 7 in, 2 out]
                    n190 = case shown="True" w415 {
                      tunnel: w417 -> [_ w422]
                      tunnel: w414 -> [_ w421]
                      tunnel: w412 -> [_ w420]
                      frame False {
                      }
                      frame True {
                        n191 = call <vilib>:"Q.Enqueue Task.vi"("Data1"=w422, "Task Name"=w420, "Q In"=w421) -> ()  [unwired: 7 in, 2 out]
                      }
                    }
                  }
                  frame True {
                  }
                }
                n192 = call <vilib>:"Scheduler.AddTask.vi"("Interval(s)"=0.1, "Task Name"=w406, "Sched Name"=w406, "Q In"=w405) -> ()  [unwired: 6 in, 2 out]
              }
              frame Error {
                n193 = call <vilib>:"Scheduler.Delete Task.vi"("Sched Name"="Serial Port - Read" ("Name"), "Q In"=w426) -> ("Q Out"=w423:refnum<queue>)  [unwired: 8 in, 1 out]
                n194 = call <vilib>:"Q.Enqueue Task.vi"("Task Name"="Update Cnct Ctrls", "Q In"=w423) -> ()  [unwired: 8 in, 2 out]
              }
            }
          }
          frame "Serial Port - Query" {
            n195 = Variant To Data(type=string[] [], Variant=w431) -> (data=w429:string[], error out=w430:errorcluster)  [unwired: 1 in]
            n196 = case shown="No Error" w430 {
              selector: w430 -> [w446 w543]
              tunnel: [w445 w542] -> _
              tunnel: [w444 w537] -> w435
              tunnel: w436 -> [w443 w537]
              tunnel: w433 -> [_ w540]
              tunnel: w434 -> [w442 _]
              tunnel: w429 -> [w441 _]
              tunnel: w428 -> [w440 _]
              tunnel: w437 -> [w439 _]
              frame No Error {
                n197 = while {
                  shift-right: [w455] -> w444
                  shift-left: w443 -> [w456]
                  shift-right: [w457] -> w445
                  shift-left: w446 -> [w458]
                  shift-right: [w459] -> _
                  shift-left: "Action" -> [w460]
                  tunnel: w442 -> [w453]
                  tunnel: w441 -> [w452]
                  tunnel: w440 -> [w451]
                  tunnel: w439 -> [w450]
                  shift-right: [w449] -> _
                  shift-left: "" -> [w448]
                  stop <- w454 stop-if-true
                  n198 = case shown="\"Action\"" w460 {
                    tunnel: ["Error Check" "Return" _] -> w459
                    tunnel: w458 -> [_ w504 w519]
                    tunnel: [w485 w502 w519] -> w457
                    tunnel: w456 -> [w491 w505 w521]
                    tunnel: [w490 w505 w520] -> w455
                    tunnel: [_ _ TRUE] -> w454
                    tunnel: w453 -> [w461 w503 _]
                    tunnel: w452 -> [w475 _ _]
                    tunnel: w451 -> [_ _ w522]
                    tunnel: w450 -> [w482 _ _]
                    tunnel: [w464 w501 _] -> w449
                    tunnel: w448 -> [_ w501 w518]
                    frame "Action" {
                      n199 = Index Array(array=w475) -> (element #1=w474:string, element #2=w473:string, element #3=w477:string)  [unwired: 3 in]
                      n200 = local read "TermChar"() -> (w481:string)
                      n201 = Decimal String To Number(string=w477, default (0L)=u32 0) -> (number=w476:u32)  [unwired: 1 in, 1 out]
                      n202 = Unbundle By Name(w491) -> ("SerialPort"=w493:refnum<class "SerialPort.lvclass">)
                      n203 = Concatenate Strings(w474, w481) -> (w465:string)
                      n204 = In Range and Coerce(upper limit=u32 5000, x=w476, lower limit=u32 1000) -> (coerced(x)=w471:u32)  [unwired: 1 out]
                      n205 = call "SerialPort.Query.vi"("TimeOut"=w471, "Term Str"=w473, "Cmd"=w465, "SerialPort in"=w493) -> ("error out"=w485:errorcluster, "Response"=w463:string, "Made Connection"=w462:bool, "SerialPort out"=w492:refnum<class "SerialPort.lvclass">, "Dur_ms"=→"Q Dur ms":u32)  [unwired: 3 in]
                      n206 = Bundle By Name(cluster=w491, "SerialPort"=w492) -> (w490:T14)
                      n207 = case shown="True" w462 {
                        tunnel: w461 -> [_ w496]
                        frame False {
                        }
                        frame True {
                          n208 = call <vilib>:"Q.Enqueue Task.vi"("Task Name"="Update Cnct Ctrls" ("Name"), "Q In"=w496) -> ()  [unwired: 8 in, 2 out]
                        }
                      }
                      n209 = Unbundle By Name(w490) -> ("Parent Tasks.Event"=w488:string)
                      n210 = Unbundle By Name(w482) -> ("Cfg.Is Child?"=w487:bool, "Cfg.Parent Q"=w489:refnum<queue>)
                      n211 = Unbundle By Name(w482) -> ("Log"=w484:refnum<class "Event Notification.lvclass">)
                      n212 = Concatenate Strings(w465, w463) -> (w470:string)
                      n213 = Build Array(u8 27) -> (w468:u8[])
                      n214 = Byte Array To String(unsigned byte array=w468) -> (string=w467:string)
                      n215 = call <vilib>:"Search and Replace Pattern.vi"("string"=w463, "regular expression (\"\")"=w467) -> ("result string"=w464:string)  [unwired: 3 in, 1 out]
                      "Q Data" <- w464
                      n216 = And(x=w462, y=w487) -> (x .and. y?=w486:bool)
                      n217 = call <vilib>:"Event Notification.Status Message.vi"("Display"=FALSE, "Level"=Event_Log.Log_Level."Debug2", "Message"=w470, "Event Notification in"=w484) -> ()  [unwired: 8 in]
                      n218 = case shown="True" w486 {
                        tunnel: w489 -> [_ w499]
                        tunnel: w488 -> [_ w498]
                        frame False {
                        }
                        frame True {
                          n219 = To Variant(anything="Connected" ("Name")) -> (Variant=w500:variant)
                          n220 = call <vilib>:"Q.Enqueue Task.vi"("Data1"=w500, "Task Name"=w498, "Q In"=w499) -> ()  [unwired: 7 in, 2 out]
                        }
                      }
                    }
                    frame "Error Check" {
                      n221 = case shown="No Error" w504 {
                        selector: w504 -> [_ w517]
                        tunnel: [_ w517] -> w502
                        tunnel: w503 -> [w512 w516]
                        tunnel: w501 -> [w509 _]
                        frame No Error {
                          n222 = To Variant(anything=w509) -> (Variant=w507:variant)
                          n223 = call <vilib>:"Q.Enqueue Task.vi"("Data1"=w507, "Task Name"="Display Data" ("Name"), "Q In"=w512) -> ("Q Out"=w511:refnum<queue>)  [unwired: 7 in, 1 out]
                          n224 = call <vilib>:"Q.Enqueue Task.vi"("Task Name"="Serial Port - Read" ("Name"), "Q In"=w511) -> ()  [unwired: 8 in, 2 out]
                        }
                        frame Error {
                          n225 = call <vilib>:"Scheduler.Delete Task.vi"("Sched Name"="Serial Port - Read" ("Name"), "Q In"=w516) -> ("Q Out"=w513:refnum<queue>)  [unwired: 8 in, 1 out]
                          n226 = call <vilib>:"Q.Enqueue Task.vi"("Task Name"="Update Cnct Ctrls" ("Name"), "Q In"=w513) -> ()  [unwired: 8 in, 2 out]
                        }
                      }
                    }
                    frame "Return", Default {
                      n227 = Variant To Data(type="", Variant=w522) -> (data=w525:string, error out=w524:errorcluster)  [unwired: 1 in]
                      n228 = case shown="No Error" w524 {
                        tunnel: w521 -> [w532 w535]
                        tunnel: [w531 w535] -> w520
                        tunnel: w525 -> [w530 _]
                        tunnel: w519 -> [w529 _]
                        tunnel: w518 -> [w528 _]
                        frame No Error {
                          n229 = Unbundle By Name(w532) -> ("FunctMgr"=w534:refnum<class "FunctMgr.lvclass">)
                          n230 = To Variant(anything=w528) -> (Variant=w527:variant)
                          n231 = call "FunctMgr.Pop and Return.vi"("error in (no error)"=w529, "Data"=w527, "Ret ID"=w530, "FunctMgr in"=w534) -> ("FunctMgr out"=w533:refnum<class "FunctMgr.lvclass">)  [unwired: 5 in, 2 out]
                          n232 = Bundle By Name(cluster=w532, "FunctMgr"=w533) -> (w531:T14)
                        }
                        frame Error {
                          # "No return message ID so do nothing."
                        }
                      }
                    }
                  }
                }
              }
              frame Error {
                n233 = Format Into String(format string="Task \"%s\" received invalid data type.  Expected string.", w540) -> (resulting string=w539:string)  [unwired: 2 in, 1 out]
                n234 = call "Error.Set-Change Error Info.vi"("error in"=w543, "Description"=w539, "Cust Code(0 = no change)"=-5100 ("Code(0 = no change)"), "Set Error"=FALSE) -> ("error out"=w542:errorcluster)  [unwired: 7 in]
              }
            }
          }
          frame "Serial Port - Write" {
            n235 = Variant To Data(type="", Variant=w553) -> (data=w546:string, error out=w552:errorcluster)  [unwired: 1 in]
            n236 = case shown="No Error" w552 {
              selector: w552 -> [w562 w643]
              tunnel: [w561 w642] -> w551
              tunnel: [w560 w637] -> w550
              tunnel: w549 -> [w559 w637]
              tunnel: w548 -> [_ w640]
              tunnel: w547 -> [w558 _]
              tunnel: w546 -> [w557 _]
              tunnel: w545 -> [w556 _]
              tunnel: w544 -> [w555 _]
              frame No Error {
                n237 = while {
                  shift-right: [w569] -> w560
                  shift-left: w559 -> [w570]
                  shift-right: [w571] -> w561
                  shift-left: w562 -> [w572]
                  shift-right: [w573] -> _
                  shift-left: "Action" -> [w574]
                  tunnel: w558 -> [w567]
                  tunnel: w557 -> [w566]
                  tunnel: w556 -> [w565]
                  tunnel: w555 -> [w564]
                  stop <- w568 stop-if-true
                  n238 = case shown="\"Action\"" w574 {
                    tunnel: ["Error Check" "Return" _] -> w573
                    tunnel: w572 -> [_ w603 w621]
                    tunnel: [w582 w601 w621] -> w571
                    tunnel: w570 -> [w589 w604 w623]
                    tunnel: [w587 w604 w622] -> w569
                    tunnel: [_ _ TRUE] -> w568
                    tunnel: w567 -> [w575 w602 _]
                    tunnel: w566 -> [w588 w600 _]
                    tunnel: w565 -> [_ _ w624]
                    tunnel: w564 -> [w578 _ _]
                    frame "Action" {
                      n239 = Unbundle By Name(w589) -> ("SerialPort"=w591:refnum<class "SerialPort.lvclass">)
                      n240 = Concatenate Strings(w588, "TermChar") -> (w577:string)
                      n241 = call "SerialPort.Write.vi"("Data"=w577, "SerialPort in"=w591) -> ("error out"=w582:errorcluster, "Made Connection"=w576:bool, "SerialPort out"=w590:refnum<class "SerialPort.lvclass">)  [unwired: 6 in, 1 out]
                      n242 = Bundle By Name(cluster=w589, "SerialPort"=w590) -> (w587:T14)
                      n243 = Unbundle By Name(w587) -> ("Parent Tasks.Event"=w585:string)
                      n244 = Unbundle By Name(w578) -> ("Cfg.Is Child?"=w584:bool, "Cfg.Parent Q"=w586:refnum<queue>)
                      n245 = Unbundle By Name(w578) -> ("Log"=w581:refnum<class "Event Notification.lvclass">)
                      n246 = And(x=w576, y=w584) -> (x .and. y?=w583:bool)
                      n247 = call <vilib>:"Event Notification.Status Message.vi"("Display"=FALSE, "Level"=Event_Log.Log_Level."Debug2", "Message"=w577, "Event Notification in"=w581) -> ()  [unwired: 8 in]
                      n248 = case shown="True" w576 {
                        tunnel: w575 -> [_ w595]
                        frame False {
                        }
                        frame True {
                          n249 = call <vilib>:"Q.Enqueue Task.vi"("Task Name"="Update Cnct Ctrls" ("Name"), "Q In"=w595) -> ()  [unwired: 8 in, 2 out]
                        }
                      }
                      n250 = case shown="True" w583 {
                        tunnel: w586 -> [_ w598]
                        tunnel: w585 -> [_ w597]
                        frame False {
                        }
                        frame True {
                          n251 = To Variant(anything="Connected" ("Name")) -> (Variant=w599:variant)
                          n252 = call <vilib>:"Q.Enqueue Task.vi"("Data1"=w599, "Task Name"=w597, "Q In"=w598) -> ()  [unwired: 7 in, 2 out]
                        }
                      }
                    }
                    frame "Error Check" {
                      n253 = case shown="No Error" w603 {
                        selector: w603 -> [_ w620]
                        tunnel: [_ w620] -> w601
                        tunnel: w602 -> [w609 w619]
                        tunnel: w600 -> [w606 _]
                        frame No Error {
                          n254 = disable-structure shown="Disabled" {
                            disable-tunnel: w609 -> [w614 w615]
                            disable-tunnel: [w611 w615] -> w608
                            disable-tunnel: w606 -> [w610 _]
                            frame Disabled {
                              n255 = To Variant(anything=w610) -> (Variant=w612:variant)
                              n256 = call <vilib>:"Q.Enqueue Task.vi"("Data1"=w612, "Task Name"="Display Data" ("Name"), "Q In"=w614) -> ("Q Out"=w611:refnum<queue>)  [unwired: 7 in, 1 out]
                            }
                            frame Enabled {
                            }
                          }
                          n257 = invoke on="Write" class="Str" method="Reinit To Default"() -> ()  [unwired: 3 in, 3 out]
                          n258 = call <vilib>:"Q.Enqueue Task.vi"("Task Name"="Serial Port - Read" ("Name"), "Q In"=w608) -> ()  [unwired: 8 in, 2 out]
                        }
                        frame Error {
                          n259 = call <vilib>:"Scheduler.Delete Task.vi"("Sched Name"="Serial Port - Read" ("Name"), "Q In"=w619) -> ("Q Out"=w616:refnum<queue>)  [unwired: 8 in, 1 out]
                          n260 = call <vilib>:"Q.Enqueue Task.vi"("Task Name"="Update Cnct Ctrls" ("Name"), "Q In"=w616) -> ()  [unwired: 8 in, 2 out]
                        }
                      }
                    }
                    frame "Return", Default {
                      n261 = Variant To Data(type="", Variant=w624) -> (data=w627:string, error out=w626:errorcluster)  [unwired: 1 in]
                      n262 = case shown="No Error" w626 {
                        tunnel: w623 -> [w632 w635]
                        tunnel: [w631 w635] -> w622
                        tunnel: w627 -> [w630 _]
                        tunnel: w621 -> [w629 _]
                        frame No Error {
                          n263 = Unbundle By Name(w632) -> ("FunctMgr"=w634:refnum<class "FunctMgr.lvclass">)
                          n264 = call "FunctMgr.Pop and Return.vi"("error in (no error)"=w629, "Ret ID"=w630, "FunctMgr in"=w634) -> ("FunctMgr out"=w633:refnum<class "FunctMgr.lvclass">)  [unwired: 6 in, 2 out]
                          n265 = Bundle By Name(cluster=w632, "FunctMgr"=w633) -> (w631:T14)
                        }
                        frame Error {
                          # "No return message ID so do nothing."
                        }
                      }
                    }
                  }
                }
              }
              frame Error {
                n266 = Format Into String(format string="Task \"%s\" received invalid data type.  Expected string.", w640) -> (resulting string=w639:string)  [unwired: 2 in, 1 out]
                n267 = call "Error.Set-Change Error Info.vi"("error in"=w643, "Description"=w639, "Cust Code(0 = no change)"=-5100 ("Code(0 = no change)"), "Set Error"=FALSE) -> ("error out"=w642:errorcluster)  [unwired: 7 in]
              }
            }
          }
          frame "Serial Port - Disconnect" {
            n268 = Unbundle By Name(w647) -> ("Log"=w646:refnum<class "Event Notification.lvclass">)
            n269 = Unbundle By Name(w648) -> ("SerialPort"=w657:refnum<class "SerialPort.lvclass">)
            n270 = call <vilib>:"Event Notification.Status Message.vi"("Level"=Event_Log.Log_Level."Verbose", "Message"="Disconnected", "Event Notification in"=w646) -> ()  [unwired: 9 in]
            n271 = call "SerialPort.Disconnect.vi"("SerialPort in"=w657) -> ("error out"=w649:errorcluster, "SerialPort out"=w658:refnum<class "SerialPort.lvclass">)  [unwired: 8 in, 1 out]
            n272 = call <vilib>:"Scheduler.Delete Task.vi"("Sched Name"="Serial Port - Read" ("Name"), "Q In"=w659) -> ("Q Out"=w650:refnum<queue>)  [unwired: 8 in, 1 out]
            n273 = Bundle By Name(cluster=w648, "SerialPort"=w658) -> (w652:T14)
            n274 = call <vilib>:"Clear Errors.vi"("error in (no error)"=w649) -> ()  [unwired: 5 in, 2 out]
            n275 = call <vilib>:"Q.Enqueue Task.vi"("Task Name"="Update Cnct Ctrls", "Q In"=w650) -> ()  [unwired: 8 in, 2 out]
            n276 = Unbundle By Name(w652) -> ("Parent Tasks.Event"=w653:string)
            n277 = Unbundle By Name(w647) -> ("Cfg.Is Child?"=w655:bool, "Cfg.Parent Q"=w654:refnum<queue>)
            n278 = case shown="True" w655 {
              tunnel: w654 -> [_ w662]
              tunnel: w653 -> [_ w661]
              tunnel: [_ w660] -> _
              frame False {
              }
              frame True {
                n279 = To Variant(anything="Disconnected" ("Name")) -> (Variant=w664:variant)
                n280 = call <vilib>:"Q.Enqueue Task.vi"("Data1"=w664, "Task Name"=w661, "Q In"=w662) -> ("error out"=w660:errorcluster)  [unwired: 7 in, 1 out]
              }
            }
          }
          frame "Display Data" {
            n281 = Variant To Data(type="", Variant=w677) -> (data=w665:string)  [unwired: 1 in, 1 out]
            n282 = Unbundle By Name(w667) -> ("Log"=w672:string)
            n283 = Concatenate Strings(w672, w665) -> (w674:string)
            n284 = String Length(string=w674) -> (length=w675:i32)
            n285 = Greater?(x=w675, y="Log Size (Chars)") -> (0:w676:bool)
            n286 = case shown="False" w676 {
              tunnel: w674 -> [w685 w688]
              tunnel: [w685 w687] -> w668
              tunnel: w675 -> [_ w686]
              tunnel: [TRUE _] -> w670
              frame False {
              }
              frame True {
                n287 = Multiply(x=w686, y=0.25) -> (x*y=w690:dbl)
                n288 = String Subset(string=w688, offset (0)=w690) -> (substring=w687:string)  [unwired: 1 in]
              }
            }
            n289 = Or(x=w670, y="Auto Scroll") -> (x .or. y?=w671:bool)
            n290 = Bundle By Name(cluster=w667, "Log"=w668) -> (w666:T14)
            n291 = case shown="True" w671 {
              tunnel: w668 -> [_ w680]
              frame False {
              }
              frame True {
                "Log" <- w680
              }
            }
            n292 = case shown="True" "Auto Scroll" {
              tunnel: w668 -> [_ w681]
              frame False {
              }
              frame True {
                n293 = String Length(string=w681) -> (length=w683:i32)
                n294 = property on="Auto Scroll" class="Bool (strict)"("BoolText.BGColor"=u32 16777216 ("Boolean Text.Text Colors:Text Color")) -> ()  [unwired: 2 in, 2 out]
                n295 = property on="Log" class="Str"("Text.Scroll Position"=w683) -> ()  [unwired: 2 in, 2 out]
              }
            }
          }
          frame "Save Log to File" {
            w694 = T16 2 items=["User Home"=0, "User Desktop"=1, "User Documents"=2, "User Application Data"=3, "User Preferences"=4, "User Temporary"=5, "Public Documents"=6, "Public Application Data"=7, "Public Preferences"=8, "Public Cache"=13, "System Core Libraries"=9, "System Installed Libraries"=10, "Application Files"=11, "Boot Volume Root"=12] ("system directory type")
            n296 = Format Date/Time String(time format string (%c)="Serial Port log, %H%M%S_%m%d%Y.txt" ("prompt (Choose or enter file path)")) -> (date/time string=w692:string)  [unwired: 2 in]
            n297 = call <vilib>:"Get System Directory.vi"("system directory type"=w694) -> ("system directory"=w693:path)  [unwired: 10 in]
            n298 = Build Path(base path=w693, name or relative path=w692) -> (appended path=w691:path)
            n299 = Unbundle By Name(w705) -> ("Log"=w698:string)
            n300 = Open/Create/Replace File(file path (use dialog)=w691, operation (0:open)=T10."replace or create") -> (refnum out=w701:refnum<file>, cancelled=w696:bool, error out=w704:errorcluster)  [unwired: 4 in]
            n301 = Write to Text File(file (use dialog)=w701, text=w698, error in=w704) -> (refnum out=w702:refnum<file>, error out=w703:errorcluster)  [unwired: 1 in, 1 out]
            n302 = Close File(refnum=w702, error in=w703) -> (path=w700:path, error out=w699:errorcluster)
            n303 = case shown="False" w696 {
              tunnel: w700 -> [w708 _]
              tunnel: w699 -> [w707 _]
              frame False {
                n304 = call <vilib>:"File.Open File or Folder.vi"("Error In"=w707, "Path"=w708) -> ()  [unwired: 9 in, 1 out]
              }
              frame True {
              }
            }
          }
          frame "Return" {
            n305 = Variant To Data(type="", Variant=w710) -> (data=w715:string, error out=w714:errorcluster)  [unwired: 1 in]
            n306 = case shown="No Error" w714 {
              selector: w714 -> [_ w727]
              tunnel: w715 -> [w724 _]
              tunnel: [w722 w727] -> w711
              tunnel: w713 -> [w721 w726]
              tunnel: [w720 w726] -> w712
              tunnel: w709 -> [w718 _]
              frame No Error {
                n307 = Unbundle By Name(w721) -> ("FunctMgr"=w725:refnum<class "FunctMgr.lvclass">, "Local Error"=w719:errorcluster)
                n308 = call "FunctMgr.Pop and Return.vi"("error in (no error)"=w719, "Data"=w718, "Ret ID"=w724, "FunctMgr in"=w725) -> ("error out"=w722:errorcluster, "FunctMgr out"=w723:refnum<class "FunctMgr.lvclass">)  [unwired: 5 in, 1 out]
                n309 = Bundle By Name(cluster=w721, "FunctMgr"=w723) -> (w720:T14)
              }
              frame Error {
                # "Can't Return.  Invalid ID."
              }
            }
          }
          frame "Status" {
            n310 = Variant To Data(type="", Variant=w731) -> (data=w733:string, error out=w732:errorcluster)  [unwired: 1 in]
            n311 = case shown="No Error" w732 {
              selector: w732 -> [_ w739]
              tunnel: w730 -> [w738 _]
              tunnel: w729 -> [_ _]
              tunnel: w733 -> [w736 _]
              tunnel: [_ w739] -> w728
              frame No Error {
                # "Received from Child\nOnly write to status indicator (not event log)\nChild already recorded to event log."
                n312 = Unbundle By Name(w738) -> ("Log"=w737:refnum<class "Event Notification.lvclass">)
                n313 = call <vilib>:"Event Notification.Status Message.vi"("Log"=FALSE, "Message"=w736, "Event Notification in"=w737) -> ()  [unwired: 9 in]
              }
              frame Error {
              }
            }
          }
          frame Default {
            n314 = call <vilib>:"Module.Default Tasks.vi"("Sys"=w745, "error in"=w741, "Data2"=w742, "Data1"=w743, "Sub"=w744) -> ("error out"=w740:errorcluster)  [unwired: 5 in, 1 out]
          }
        }
      }
      frame "Function" {
        # "Return by default"
        n315 = case shown="\"Write\"" w755 {
          selector: w755 -> [_ w784 w806 w838 _ _ _ w891 w922 _ w969]
          tunnel: w759 -> [w773 w790 w812 w844 w868 w881 w886 w898 w928 w956 w973]
          tunnel: w758 -> [w772 w787 w809 w841 w865 w878 w885 w894 w925 w951 w974]
          tunnel: [w773 w790 w812 w844 w868 w881 w886 w898 w928 w956 w973] -> w757
          tunnel: [w772 w786 w808 w840 w865 w877 w885 w893 w924 w950 w974] -> w756
          tunnel: w754 -> [w770 w789 w811 w842 _ w879 _ w895 w926 w947 _]
          tunnel: w753 -> [w771 w788 w810 w833 w866 w870 w883 w888 w919 _ w970]
          tunnel: w752 -> [_ _ _ _ _ _ _ _ _ _ _]
          tunnel: w750 -> [_ w780 w802 w834 _ w880 _ w897 w927 w948 w968]
          tunnel: [w766 w783 w805 w837 _ _ _ w890 w921 w953 w967] -> w749
          tunnel: [_ _ _ _ _ _ _ _ _ _ variant] -> w748
          tunnel: [FALSE w782 w804 w836 _ TRUE _ w889 w920 TRUE FALSE] -> w747
          frame "Lock Controls" {
            n316 = Variant To Data(type=FALSE, Variant=w770) -> (data=w768:bool, error out=w767:errorcluster)  [unwired: 1 in]
            n317 = case shown="No Error" w767 {
              selector: w767 -> [_ w778]
              tunnel: w771 -> [w775 _]
              tunnel: w768 -> [w774 _]
              tunnel: [_ w778] -> w766
              frame No Error {
                n318 = To Variant(anything=w774) -> (Variant=w777:variant)
                n319 = call <vilib>:"Q.Enqueue Task.vi"("Data1"=w777, "Task Name"="Lock Test Controls", "Q In"=w775) -> ()  [unwired: 7 in, 2 out]
              }
              frame Error {
              }
            }
          }
          frame "Set Parent Task Names" {
            n320 = Variant To Data(type=T8 {"Rcv"="Serial Port - Read", "Event"="Serial Port - Events"} ("Parent Tasks"), Variant=w789) -> (data=w781:T8, error out=w785:errorcluster)  [unwired: 1 in]
            n321 = case shown="Error" w785 {
              selector: w785 -> [_ w795]
              tunnel: w789 -> [_ _]
              tunnel: w788 -> [_ w798]
              tunnel: w787 -> [w793 w800]
              tunnel: [w792 w800] -> w786
              tunnel: w784 -> [_ w797]
              tunnel: [_ w796] -> w783
              tunnel: [_ FALSE] -> w782
              tunnel: w781 -> [w791 _]
              tunnel: w780 -> [_ w794]
              frame No Error {
                n322 = Bundle By Name(cluster=w793, "Parent Tasks"=w791) -> (w792:T14)
              }
              frame Error {
                n323 = call <vilib>:"SeqMgr.Error, Build Parameter Error Message.vi"("error in"=w795, "Data2"=w794, "Funct Name"=w797, "Local Q"=w798) -> ("error out"=w796:errorcluster)  [unwired: 7 in]
              }
            }
          }
          frame "Config Port" {
            n324 = Variant To Data(type=T11 {"Port Name"="", "Config"={"Baud Rate (115200)"=0, "Data Bits (8)"=0, "Parity (0:none)"=enum."None", "Stop Bits (10: 1 bit)"=0, "Flow Control (0:none)"=enum."None", "Enable Term Char (T)"=FALSE, "Term Char(0xA = '\\n' = LF) "=0}, "Port Timeout ms (3000)"=0} ("output cluster"), Variant=w811) -> (data=w803:T11, error out=w807:errorcluster)  [unwired: 1 in]
            n325 = case shown="No Error" w807 {
              selector: w807 -> [_ w827]
              tunnel: w811 -> [_ _]
              tunnel: w810 -> [w818 w830]
              tunnel: w809 -> [w825 w832]
              tunnel: [w824 w832] -> w808
              tunnel: w806 -> [_ w829]
              tunnel: [w813 w828] -> w805
              tunnel: [FALSE FALSE] -> w804
              tunnel: w803 -> [w817 _]
              tunnel: w802 -> [_ w826]
              frame No Error {
                n326 = local read "COM Port"() -> (w814:refnum<visa-resource-name>)
                n327 = Unbundle(w817) -> ("Config"=w815:T1, "Port Timeout ms (3000)"=w816:u32)  [unwired: 1 out]
                n328 = Unbundle By Name(w825) -> ("SerialPort"=w821:refnum<class "SerialPort.lvclass">)
                n329 = control-ref of="State"() -> (w820:refnum<vi>)
                n330 = call "SerialPort.Config_All.vi"("Timeout ms (3sec)"=w816, "State Ctrl Ref"=w820, "Config"=w815, "Com Port"=w814, "SerialPort in"=w821) -> ("error out"=w813:errorcluster, "SerialPort out"=w822:refnum<class "SerialPort.lvclass">)  [unwired: 5 in]
                n331 = call <vilib>:"Q.Enqueue Task.vi"("Task Name"="Update Cnct Ctrls", "Q In"=w818) -> ()  [unwired: 8 in, 2 out]
                n332 = Bundle By Name(cluster=w825, "SerialPort"=w822) -> (w824:T14)
              }
              frame Error {
                n333 = call <vilib>:"SeqMgr.Error, Build Parameter Error Message.vi"("error in"=w827, "Data2"=w826, "Funct Name"=w829, "Local Q"=w830) -> ("error out"=w828:errorcluster)  [unwired: 7 in]
              }
            }
          }
          frame "Set Port" {
            n334 = Variant To Data(type="", Variant=w842) -> (data=w835:string, error out=w839:errorcluster)  [unwired: 1 in]
            n335 = case shown="No Error" w839 {
              selector: w839 -> [_ w858]
              tunnel: w842 -> [_ _]
              tunnel: w833 -> [w846 w861]
              tunnel: w841 -> [w856 w863]
              tunnel: [w855 w863] -> w840
              tunnel: w838 -> [_ w860]
              tunnel: [w845 w859] -> w837
              tunnel: [TRUE FALSE] -> w836
              tunnel: w835 -> [w848 _]
              tunnel: w834 -> [_ w857]
              frame No Error {
                n336 = local read "Timeout ms (3sec)"() -> (w849:u32)
                n337 = Unbundle By Name(w856) -> ("SerialPort"=w852:refnum<class "SerialPort.lvclass">)
                n338 = local read "Config"() -> (w850:T1)
                n339 = control-ref of="State"() -> (w851:refnum<vi>)
                n340 = call "SerialPort.Config_All.vi"("Timeout ms (3sec)"=w849, "State Ctrl Ref"=w851, "Config"=w850, "Com Port"=w848, "SerialPort in"=w852) -> ("error out"=w845:errorcluster, "SerialPort out"=w853:refnum<class "SerialPort.lvclass">)  [unwired: 5 in]
                n341 = call <vilib>:"Q.Enqueue Task.vi"("Task Name"="Update Cnct Ctrls", "Q In"=w846) -> ()  [unwired: 8 in, 2 out]
                n342 = Bundle By Name(cluster=w856, "SerialPort"=w853) -> (w855:T14)
              }
              frame Error {
                n343 = call <vilib>:"SeqMgr.Error, Build Parameter Error Message.vi"("error in"=w858, "Data2"=w857, "Funct Name"=w860, "Local Q"=w861) -> ("error out"=w859:errorcluster)  [unwired: 7 in]
              }
            }
          }
          frame "AutoFindPort" {
            n344 = call <vilib>:"Q.Enqueue Task.vi"("Task Name"="Serial Port - Auto Find", "Q In"=w866) -> ()  [unwired: 8 in, 2 out]
            n345 = local write "Auto Find Port"(TRUE ("Auto Find Port")) -> ()
          }
          frame "Connect" {
            n346 = call "Error.Clear.vi"("Q In"=w870) -> ("Q Out"=w869:refnum<queue>)  [unwired: 9 in, 1 out]
            n347 = Unbundle By Name(w878) -> ("FunctMgr"=w875:refnum<class "FunctMgr.lvclass">)
            n348 = call "FunctMgr.Push Return Info.vi"("Ret Info"=w880, "FunctMgr in"=w875) -> ("Ret ID"=w873:string, "FunctMgr out"=w874:refnum<class "FunctMgr.lvclass">)  [unwired: 6 in, 2 out]
            n349 = To Variant(anything=w873) -> (Variant=w871:variant)
            n350 = Bundle By Name(cluster=w878, "FunctMgr"=w874) -> (w877:T14)
            n351 = call <vilib>:"Q.Enqueue Task.vi"("Data2"=w871, "Data1"=w879, "Task Name"="Serial Port - Connect" ("Name"), "Q In"=w869) -> ()  [unwired: 6 in, 2 out]
          }
          frame "Disconnect" {
            n352 = call "Error.Clear.vi"("Q In"=w883) -> ("Q Out"=w882:refnum<queue>)  [unwired: 9 in, 1 out]
            n353 = call <vilib>:"Q.Enqueue Task.vi"("Task Name"="Serial Port - Disconnect" ("Name"), "Q In"=w882) -> ()  [unwired: 8 in, 2 out]
          }
          frame "Write" {
            n354 = call "Error.Clear.vi"("Q In"=w888) -> ("Q Out"=w887:refnum<queue>)  [unwired: 9 in, 1 out]
            n355 = Variant To Data(type="", Variant=w895) -> (error out=w892:errorcluster)  [unwired: 1 in, 1 out]
            n356 = case shown="No Error" w892 {
              selector: w892 -> [_ w910]
              tunnel: w897 -> [w900 w912]
              tunnel: w895 -> [w906 _]
              tunnel: w887 -> [w903 w914]
              tunnel: w894 -> [w902 w916]
              tunnel: [w901 w916] -> w893
              tunnel: w891 -> [_ w913]
              tunnel: [_ w911] -> w890
              tunnel: [TRUE FALSE] -> w889
              frame No Error {
                n357 = Unbundle By Name(w902) -> ("FunctMgr"=w909:refnum<class "FunctMgr.lvclass">)
                n358 = call "FunctMgr.Push Return Info.vi"("Ret Info"=w900, "FunctMgr in"=w909) -> ("Ret ID"=w907:string, "FunctMgr out"=w908:refnum<class "FunctMgr.lvclass">)  [unwired: 6 in, 2 out]
                n359 = To Variant(anything=w907) -> (Variant=w904:variant)
                n360 = Bundle By Name(cluster=w902, "FunctMgr"=w908) -> (w901:T14)
                n361 = call <vilib>:"Q.Enqueue Task.vi"("Data2"=w904, "Data1"=w906, "Task Name"="Serial Port - Write" ("Name"), "Q In"=w903) -> ()  [unwired: 6 in, 2 out]
              }
              frame Error {
                n362 = call <vilib>:"SeqMgr.Error, Build Parameter Error Message.vi"("error in"=w910, "Data2"=w912, "Funct Name"=w913, "Local Q"=w914) -> ("error out"=w911:errorcluster)  [unwired: 7 in]
              }
            }
          }
          frame "Query" {
            n363 = call "Error.Clear.vi"("Q In"=w919) -> ("Q Out"=w918:refnum<queue>)  [unwired: 9 in, 1 out]
            n364 = Variant To Data(type=string[] [], Variant=w926) -> (error out=w923:errorcluster)  [unwired: 1 in, 1 out]
            n365 = case shown="No Error" w923 {
              selector: w923 -> [_ w940]
              tunnel: w927 -> [w930 w942]
              tunnel: w926 -> [w936 _]
              tunnel: w918 -> [w933 w944]
              tunnel: w925 -> [w932 w946]
              tunnel: [w931 w946] -> w924
              tunnel: w922 -> [_ w943]
              tunnel: [_ w941] -> w921
              tunnel: [TRUE FALSE] -> w920
              frame No Error {
                n366 = Unbundle By Name(w932) -> ("FunctMgr"=w939:refnum<class "FunctMgr.lvclass">)
                n367 = call "FunctMgr.Push Return Info.vi"("Ret Info"=w930, "FunctMgr in"=w939) -> ("Ret ID"=w937:string, "FunctMgr out"=w938:refnum<class "FunctMgr.lvclass">)  [unwired: 6 in, 2 out]
                n368 = To Variant(anything=w937) -> (Variant=w934:variant)
                n369 = Bundle By Name(cluster=w932, "FunctMgr"=w938) -> (w931:T14)
                n370 = call <vilib>:"Q.Enqueue Task.vi"("Data2"=w934, "Data1"=w936, "Task Name"="Serial Port - Query" ("Name"), "Q In"=w933) -> ()  [unwired: 6 in, 2 out]
              }
              frame Error {
                n371 = call <vilib>:"SeqMgr.Error, Build Parameter Error Message.vi"("error in"=w940, "Data2"=w942, "Funct Name"=w943, "Local Q"=w944) -> ("error out"=w941:errorcluster)  [unwired: 7 in]
              }
            }
          }
          frame "Return" {
            n372 = Variant To Data(type="", Variant=w948) -> (data=w954:string, error out=w949:errorcluster)  [unwired: 1 in]
            n373 = case shown="No Error" w949 {
              selector: w949 -> [_ w966]
              tunnel: w954 -> [w963 _]
              tunnel: [w961 w966] -> w953
              tunnel: w951 -> [w960 w965]
              tunnel: [w959 w965] -> w950
              tunnel: w947 -> [w957 _]
              frame No Error {
                n374 = Unbundle By Name(w960) -> ("FunctMgr"=w964:refnum<class "FunctMgr.lvclass">, "Local Error"=w958:errorcluster)
                n375 = call "FunctMgr.Pop and Return.vi"("error in (no error)"=w958, "Data"=w957, "Ret ID"=w963, "FunctMgr in"=w964) -> ("error out"=w961:errorcluster, "FunctMgr out"=w962:refnum<class "FunctMgr.lvclass">)  [unwired: 5 in, 1 out]
                n376 = Bundle By Name(cluster=w960, "FunctMgr"=w962) -> (w959:T14)
              }
              frame Error {
                # "Can't Return.  Invalid ID."
              }
            }
          }
          frame Default {
            n377 = call <vilib>:"SeqMgr.Error, Build Function Name Error Message.vi"("Data2"=w968, "Funct_Seq Name"=w969, "Local Q"=w970) -> ("error out"=w967:errorcluster)  [unwired: 8 in]
          }
        }
        n378 = case shown="False" w747 {
          tunnel: [w763 w764] -> w751
          tunnel: w750 -> [w762 _]
          tunnel: w749 -> [w761 w764]
          tunnel: w748 -> [w760 _]
          frame False {
            n379 = call <vilib>:"Q.Return Function Data.vi"("error in"=w761, "Data2"=w762, "Ret Data"=w760) -> ("error out"=w763:errorcluster)  [unwired: 8 in]
          }
          frame True {
          }
        }
      }
      frame "App" {
        n380 = case shown="\"Set Logging Level\"" w982 {
          tunnel: w981 -> [_ _]
          tunnel: w980 -> [_ w994]
          tunnel: w979 -> [_ _]
          tunnel: w978 -> [w984 w991]
          tunnel: w977 -> [w983 w993]
          tunnel: [w984 w992] -> w976
          tunnel: [w983 w993] -> w975
          frame Default {
          }
          frame "Set Logging Level" {
            n381 = Variant To Data(type=Event_Log.Log_Level."Normal" ("Log Level"), Variant=w994) -> (data=w987:T2)  [unwired: 1 in, 1 out]
            n382 = local read "Logging Level"() -> (w986:T2)
            n383 = Unbundle By Name(w991) -> ("Log"=w989:refnum<class "Event Notification.lvclass">)
            n384 = Not Equal?(x=w987, y=w986) -> (x != y?=w985:bool)
            n385 = call <vilib>:"Event Notification.Set Logging Level.vi"("Log Level"=w987, "Event Notification in"=w989) -> ("Event Notification out"=w990:refnum<class "Event Notification.lvclass">)  [unwired: 9 in]
            n386 = case shown="True" w985 {
              tunnel: w987 -> [_ w995]
              frame False {
              }
              frame True {
                n387 = local write "Logging Level"(w995) -> ()
              }
            }
            n388 = Bundle By Name(cluster=w991, "Log"=w990) -> (w992:T7)
          }
        }
      }
      frame "Error", Default {
        n389 = case shown="\"Error\"" w1003 {
          selector: w1003 -> [_ w1058]
          tunnel: [_ w1059] -> w1004
          tunnel: w1002 -> [w1013 _]
          tunnel: w1001 -> [w1011 _]
          tunnel: w1000 -> [w1012 _]
          tunnel: w999 -> [w1010 _]
          tunnel: w997 -> [w1007 w1057]
          tunnel: w998 -> [w1008 _]
          tunnel: [w1006 w1057] -> w996
          frame "Error" {
            n390 = case shown="\"Error\"" w1012 {
              tunnel: w1013 -> [_ w1055 _]
              tunnel: w1011 -> [w1051 _ _]
              tunnel: [w1051 w1053 _] -> w1005
              tunnel: w1010 -> [w1050 w1052 w1056]
              tunnel: [w1050 w1052 w1056] -> w1009
              frame Default {
              }
              frame "Error" {
                n391 = Variant To Data(type=errorcluster {"status"=FALSE, "code"=0, "source"=""} ("error constant"), Variant=w1055) -> (data=w1053:errorcluster)  [unwired: 1 in, 1 out]
              }
              frame "Clear" {
              }
            }
            n392 = case shown="No Error" w1005 {
              selector: w1005 -> [_ w1029]
              tunnel: w1009 -> [_ w1042]
              tunnel: w1008 -> [w1015 w1027]
              tunnel: w1007 -> [w1018 w1036]
              tunnel: [w1017 w1035] -> w1006
              frame No Error {
                # "Clear Local Errors"
                n393 = Unbundle By Name(w1018) -> ("Local Error"=w1020:errorcluster)
                n394 = Unbundle By Name(w1015) -> ("Log"=w1014:refnum<class "Event Notification.lvclass">)
                n395 = case shown="Error" w1020 {
                  tunnel: w1014 -> [_ w1023]
                  frame No Error {
                  }
                  frame Error {
                    n396 = call <vilib>:"Event Notification.Status Message.vi"("Level"=Event_Log.Log_Level."Verbose", "Message"="Cleared Errors", "Event Notification in"=w1023) -> ()  [unwired: 9 in]
                  }
                }
                n397 = control-ref of="Error Status"() -> (w1016:refnum<vi>)
                n398 = invoke on="Error" class="Clust (strict)" method="Reinit To Default"() -> ()  [unwired: 3 in, 3 out]
                n399 = call <vilib>:"Status.Simple Text Status Indicator.vi"("Status TextBox"=w1016) -> ()  [unwired: 10 in, 1 out]
                n400 = Bundle By Name(cluster=w1018, "Local Error"=errorcluster {"status"=FALSE, "code"=0, "source"=""}) -> (w1017:T14)
              }
              frame Error {
                # "Record Error"
                # "Disable"
                # "If is child, forward error"
                n401 = Unbundle By Name(w1036) -> ("Local Error"=w1034:errorcluster)
                n402 = Unbundle By Name(w1027) -> ("Log"=w1026:refnum<class "Event Notification.lvclass">)
                n403 = Unbundle By Name(w1029) -> ("code"=w1040:i32, "source"=w1039:string)
                n404 = Format Into String(format string="ERROR!!! Code: %d, Desc: %s", w1040, w1039) -> (resulting string=w1025:string)  [unwired: 2 in, 1 out]
                n405 = call <vilib>:"Q.Enqueue Task.vi"("Task Name"="Serial Port - Disconnect" ("Name"), "Q In"=w1042) -> ()  [unwired: 8 in, 2 out]
                n406 = control-ref of="Error Status"() -> (w1028:refnum<vi>)
                n407 = Merge Errors(w1034, w1029) -> (w1033:errorcluster)
                n408 = call <vilib>:"Event Notification.Status Message with Error In.vi"("Type"=Event_Log.Notification_Type."Error", "Message"=w1025, "Event Notification in"=w1026) -> ()  [unwired: 9 in]
                n409 = call <vilib>:"Status.Simple Text Status Indicator.vi"("error in"=w1029, "Status TextBox"=w1028) -> ()  [unwired: 9 in, 1 out]
                n410 = Unbundle By Name(w1036) -> ("Parent Tasks.Event"=w1038:string)
                n411 = Unbundle By Name(w1027) -> ("Cfg.Is Child?"=w1032:bool, "Cfg.Parent Q"=w1037:refnum<queue>)
                n412 = Bundle By Name(cluster=w1036, "Local Error"=w1033) -> (w1035:T14)
                n413 = And(x=FALSE, y=w1032) -> (x .and. y?=w1031:bool)
                n414 = case shown="True" w1031 {
                  tunnel: w1037 -> [_ w1049]
                  tunnel: w1038 -> [_ w1048]
                  tunnel: w1029 -> [_ w1045]
                  frame False {
                  }
                  frame True {
                    n415 = To Variant(anything="Error") -> (Variant=w1047:variant)
                    n416 = To Variant(anything=w1045) -> (Variant=w1044:variant)
                    n417 = call <vilib>:"Q.Enqueue Task.vi"("Data2"=w1044, "Data1"=w1047, "Task Name"=w1048, "Q In"=w1049) -> ()  [unwired: 6 in, 2 out]
                  }
                }
                "Error" <- w1029
              }
            }
          }
          frame Default {
            n418 = Concatenate Strings("Undefined State: \"", w1058, "\".") -> (w1060:string)
            n419 = Bundle By Name(cluster=errorcluster {"status"=TRUE, "code"=-5000, "source"=""} ("error constant"), "source"=w1060) -> (w1059:errorcluster)
          }
        }
      }
      frame "Exit" {
        # "This connection is made to not close\n the module until exit tasks are done."
        n420 = stacked-sequence {
          tunnel: w1065 -> [w1069 w1072]
          tunnel: [errorcluster {"status"=FALSE, "code"=0, "source"=""} ("error constant") _] -> w1064
          frame #0 {
            # "Close connection to instruments"
            n421 = Unbundle By Name(w1069) -> ("SerialPort"=w1070:refnum<class "SerialPort.lvclass">)
            n422 = call "SerialPort.Disconnect.vi"("SerialPort in"=w1070) -> ()  [unwired: 8 in, 3 out]
          }
          frame #1 {
            # "Leave error not connected\nIgnore errors"
            # "Send Exit command to child modules"
            n423 = Unbundle By Name(w1072) -> ("App.Child Modules"=w1073:cluster{"VI Ref":refnum<vi>, "Name":string}[])
            n424 = for {
              tunnel: w1073 -> [w1076] mode=indexing
              tunnel: [w1074] -> _ mode=indexing
              n425 = Unbundle By Name(w1076) -> ("Name"=w1075:string)
              n426 = call <vilib>:"Q.Enqueue Exit.vi"("Q Name"=w1075) -> ("error out"=w1074:errorcluster)  [unwired: 9 in, 1 out]
            }
          }
        }
        n427 = call <vilib>:"Module.Destructor.vi"("error in"=w1064, "Sys"=w1066) -> ("error out"=w1068:errorcluster)  [unwired: 9 in]
      }
    }
  }
  n428 = while "Event Loop" {
    tunnel: w9 -> [w1083]
    shift-right: [w1077] -> _
    shift-left: w6 -> [w1079]
    shift-right: [w1078] -> _
    shift-left: w5 -> [w1080]
    stop <- w1084 stop-if-true
    n429 = Unbundle By Name(w1083) -> ("Stop.Ref"=w1082:refnum<event-registration>, "Main Q"=w1081:refnum<queue>)
    n430 = event shown="[14] \"Write\": Key Down" {
      selector: w1082 -> [_ _ _ _ _ _ _ _ _ _ _ _ _ _ _ _ _]
      dyn-events: _ -> [_ _ _ _ _ _ _ _ _ _ _ _ _ _ _ _ _]
      timeout: _ -> [_ _ _ _ _ _ _ _ _ _ _ _ _ _ _ _ _]
      tunnel: [w1089 _ _ w1113 TRUE _ _ _ _ _ _ _ _ _ _ _ _] -> w1084
      tunnel: w1083 -> [w1088 _ _ w1111 _ _ _ _ _ _ _ _ _ _ _ _ _]
      tunnel: w1081 -> [w1091 w1103 _ w1112 _ _ w1141 w1147 w1157 w1161 w1165 w1168 w1176 w1181 w1183 _ w1226]
      tunnel: w1080 -> [w1086 w1101 w1105 w1108 w1135 w1138 w1140 w1146 w1156 w1160 w1164 w1170 w1178 w1180 w1188 w1221 w1229]
      tunnel: w1079 -> [w1085 w1100 w1104 w1107 w1134 w1137 w1139 w1145 w1155 w1159 w1163 w1169 w1177 w1179 w1184 w1220 w1228]
      tunnel: [w1086 w1101 w1105 w1108 w1135 w1138 w1140 w1146 w1156 w1160 w1164 w1170 w1178 w1180 w1187 w1221 w1229] -> w1078
      tunnel: [w1085 w1100 w1104 w1107 w1134 w1137 w1139 w1145 w1155 w1159 w1163 w1169 w1177 w1179 w1186 w1220 w1228] -> w1077
      event Panel Close? {
        n431 = event-data() -> ()  [unwired: 1 in, 4 out]
        n432 = Unbundle By Name(w1088) -> ("Cfg.Is Child?"=w1087:bool)
        n433 = case shown="True" w1087 {
          tunnel: w1091 -> [w1094 w1097]
          tunnel: [TRUE TRUE] -> w1090
          tunnel: [TRUE FALSE] -> w1089
          tunnel: [_ w1095] -> _
          frame False {
            # "Parent - Exit"
            n434 = call <vilib>:"Q.Enqueue Exit.vi"("Q In"=w1094) -> ()  [unwired: 9 in, 2 out]
          }
          frame True {
            # "Child - Hide Panel and if was \nin a subpanel, return to subpanel."
            n435 = call <vilib>:"Module.Window, Q Task.vi"("Action"=Window.Task,_Action."Return to SubPanel()", "Q In"=w1097) -> ("error out"=w1095:errorcluster)  [unwired: 8 in, 1 out]
          }
        }
        n436 = event-data("Discard?"=w1090) -> ()  [unwired: 1 in, 1 out]
      }
      event Panel Resize {
        n437 = event-data() -> ()  [unwired: 1 in, 8 out]
        n438 = call <vilib>:"Module.Window, Q Task.vi"("Action"=Window.Task,_Action."Resize()", "Q In"=w1103) -> ()  [unwired: 8 in, 2 out]
      }
      event "Leave Maint": Value Change {
        n439 = event-data() -> ()  [unwired: 1 in, 6 out]
        n440 = local write "Main Tab"(0) -> ()
      }
      event Menu Selection (User) {
        n441 = event-data() -> ("MenuRef"=w1109:refnum<k9>, "ItemTag"=w1110:string)  [unwired: 1 in, 5 out]
        n442 = case shown="\"Help.About\"" w1110 {
          selector: w1110 -> [w1115 _ _ _ _ w1125 _ _]
          tunnel: [_ TRUE _ _ _ _ _ _] -> w1113
          tunnel: w1112 -> [_ w1118 _ w1121 _ w1129 w1131 w1133]
          tunnel: [_ _ w1120 _ _ _ _ _] -> _
          tunnel: w1111 -> [w1114 _ _ _ w1123 _ _ _]
          tunnel: w1109 -> [_ _ _ _ _ w1126 _ _]
          frame Default {
            # "Check if a help document was selected.\nIf so, open the document"
            n443 = Unbundle By Name(w1114) -> ("Docs.Tags"=w1117:string[], "Docs.Paths"=w1116:path[])
            n444 = call <vilib>:"Menu.Help, Open User Manual Items.vi"("Menu Tag Selection"=w1115, "Paths"=w1116, "Tags"=w1117) -> ()  [unwired: 8 in, 1 out]
          }
          frame "Exit" {
            n445 = call <vilib>:"Q.Enqueue Exit.vi"("Q In"=w1118) -> ()  [unwired: 9 in, 2 out]
          }
          frame "Event Log" {
            n446 = call <vilib>:"Event Log.Show.vi"() -> ("error out"=w1120:errorcluster)  [unwired: 11 in]
          }
          frame "Reset" {
            n447 = call <vilib>:"Q.Enqueue Reset.vi"("Q In"=w1121) -> ()  [unwired: 9 in, 2 out]
          }
          frame "Help.About" {
            n448 = Unbundle By Name(w1123) -> ("SW Rev"=w1122:T6)
            n449 = call <vilib>:"Help.About.vi"("SW Version"=w1122) -> ()  [unwired: 11 in]
          }
          frame "Simulate OFF", "Simulate ON" {
            n450 = call <vilib>:"Menu.Simulate, Set Menu State.vi"("Menu Tag"=w1125, "Menu Ref"=w1126) -> ("Sim ON"=w1124:bool)  [unwired: 8 in, 1 out]
            n451 = To Variant(anything=w1124) -> (Variant=w1128:variant)
            n452 = call <vilib>:"Q.Enqueue Task.vi"("Data1"=w1128, "Task Name"="Simulate", "Q In"=w1129) -> ()  [unwired: 7 in, 2 out]
          }
          frame "Show Block Diagram" {
            n453 = call <vilib>:"Module.Window, Q Task.vi"("Action"=Window.Task,_Action."Open Block Diagram()", "Q In"=w1131) -> ()  [unwired: 8 in, 2 out]
          }
          frame "Go to Maint Tab" {
            n454 = call <vilib>:"Module.Window, Q Task.vi"("Action"=Window.Task,_Action."Show Maint Tab(Bool)", "Q In"=w1133) -> ()  [unwired: 8 in, 2 out]
          }
        }
      }
      event User Event {
        n455 = event-data() -> ()  [unwired: 1 in, 5 out]
      }
      event "Clear Log": Value Change {
        n456 = event-data() -> ()  [unwired: 1 in, 6 out]
        n457 = invoke on="Log" class="Str" method="Reinit To Default"() -> ()  [unwired: 3 in, 3 out]
      }
      event "COM Port": Value Change {
        n458 = event-data() -> ()  [unwired: 1 in, 6 out]
        n459 = call <vilib>:"Q.Enqueue Task.vi"("Task Name"="Serial Port - Init" ("Name"), "Q In"=w1141) -> ()  [unwired: 8 in, 2 out]
      }
      event "Send Tab": Value Change {
        n460 = event-data() -> ()  [unwired: 1 in, 6 out]
        n461 = To Variant(anything="\t") -> (Variant=w1143:variant)
        n462 = call <vilib>:"Q.Enqueue Task.vi"("Data1"=w1143, "Task Name"="Serial Port - Write" ("Name"), "Q In"=w1147) -> ()  [unwired: 7 in, 2 out]
      }
      event "Query": Value Change {
        n463 = event-data() -> ()  [unwired: 1 in, 6 out]
        n464 = Number To Decimal String(number="Q Timeout ms") -> (decimal integer string=w1150:string)  [unwired: 1 in]
        n465 = Build Array("Q Cmd", "Q MsgEnd", w1150) -> (w1149:string[])
        n466 = To Variant(anything=w1149) -> (Variant=w1154:variant)
        n467 = call <vilib>:"Q.Enqueue Task.vi"("Data1"=w1154, "Task Name"="Serial Port - Query" ("Name"), "Q In"=w1157) -> ()  [unwired: 7 in, 2 out]
      }
      event "Timeout ms (3sec)": Value Change {
        n468 = event-data() -> ()  [unwired: 1 in, 6 out]
        n469 = call <vilib>:"Q.Enqueue Task.vi"("Task Name"="Serial Port - Set Timeout" ("Name"), "Q In"=w1161) -> ()  [unwired: 8 in, 2 out]
      }
      event "Disconnect": Value Change {
        n470 = event-data() -> ()  [unwired: 1 in, 6 out]
        n471 = call <vilib>:"Q.Enqueue Task.vi"("Task Name"="Serial Port - Disconnect" ("Name"), "Q In"=w1165) -> ()  [unwired: 8 in, 2 out]
      }
      event "Auto Find Port": Value Change {
        n472 = event-data() -> ("NewVal"=w1167:bool)  [unwired: 1 in, 5 out]
        n473 = case shown="True" w1167 {
          tunnel: w1168 -> [_ w1171]
          frame False {
          }
          frame True {
            n474 = call <vilib>:"Q.Enqueue Task.vi"("Task Name"="Serial Port - Auto Find", "Q In"=w1171) -> ()  [unwired: 8 in, 2 out]
          }
        }
      }
      event Value Change {
        n475 = event-data() -> ()  [unwired: 1 in, 6 out]
        n476 = To Variant(anything="Logging Level") -> (Variant=w1174:variant)
        n477 = call <vilib>:"Q.Enqueue Task.vi"("Data1"=w1174, "Task Name"="Set Logging Level", "Q In"=w1176) -> ()  [unwired: 7 in, 2 out]
      }
      event "Connect": Value Change {
        n478 = event-data() -> ()  [unwired: 1 in, 6 out]
        n479 = call <vilib>:"Q.Enqueue Task.vi"("Task Name"="Serial Port - Connect" ("Name"), "Q In"=w1181) -> ()  [unwired: 8 in, 2 out]
      }
      event "Write": Key Down {
        n480 = event-data() -> ("VKey"=w1185:T18)  [unwired: 1 in, 9 out]
        n481 = case shown="\"Enter\", \"Return\"" w1185 {
          selector: w1185 -> [_ _ w1206]
          tunnel: w1188 -> [w1190 w1194 w1212]
          tunnel: [w1190 w1192 w1212] -> w1187
          tunnel: [w1189 w1193 w1207] -> w1186
          tunnel: w1184 -> [w1189 _ w1214]
          tunnel: w1183 -> [_ w1191 _]
          frame "ASCII", Default {
          }
          frame "Enter", "Return" {
            n482 = stacked-sequence {
              tunnel: w1194 -> [_ w1201 _]
              tunnel: [_ w1199 _] -> w1193
              tunnel: [_ w1198 _] -> w1192
              tunnel: w1191 -> [_ _ w1204]
              frame #0 {
                n483 = property on="Write" class="Str"("Key Focus"=FALSE) -> (error out=w1195:errorcluster)  [unwired: 2 in, 1 out]
                n484 = property on="Write" class="Str"(error in=w1195, "Key Focus"=TRUE) -> ()  [unwired: 1 in, 2 out]
              }
              frame #1 {
                n485 = local read "Write"() -> (w1200:string)
                n486 = Build Array (concatenate)(w1201, w1200) -> (w1198:string[])
                n487 = Array Size(array=w1198) -> (size(s)=w1199:i32)
              }
              frame #2 {
                n488 = To Variant(anything="Write") -> (Variant=w1202:variant)
                n489 = call <vilib>:"Q.Enqueue Task.vi"("Data1"=w1202, "Task Name"="Serial Port - Write" ("Name"), "Q In"=w1204) -> ()  [unwired: 7 in, 2 out]
              }
            }
          }
          frame "Up", "Down" {
            n490 = case shown="\"Up\", Default" w1206 {
              tunnel: w1214 -> [w1216 w1218]
              tunnel: [w1215 w1217] -> w1209
              frame "Up", Default {
                n491 = Decrement(x=w1216) -> (x-1=w1215:i32)
              }
              frame "Down" {
                n492 = Increment(x=w1218) -> (x+1=w1217:i32)
              }
            }
            n493 = Array Size(array=w1212) -> (size(s)=w1211:i32)
            n494 = Decrement(x=w1211) -> (x-1=w1210:i32)
            n495 = In Range and Coerce(upper limit=w1210, x=w1209, lower limit=0) -> (coerced(x)=w1207:i32)  [unwired: 1 out]
            n496 = Index Array(array=w1212, index=w1207) -> (element=w1213:string)
            n497 = local write "Write"(w1213) -> ()
          }
        }
      }
      event "Auto Scroll": Value Change {
        n498 = event-data() -> ("NewVal"=w1219:bool)  [unwired: 1 in, 5 out]
        n499 = case shown="False" w1219 {
          frame False {
            n500 = local read "Log"() -> (w1224:string)
            n501 = String Length(string=w1224) -> (length=w1223:i32)
            n502 = property on="Auto Scroll" class="Bool (strict)"("BoolText.BGColor"=u32 16777216 ("Boolean Text.Text Colors:Text Color")) -> ()  [unwired: 2 in, 2 out]
            n503 = property on="Log" class="Str"("Text.Scroll Position"=w1223) -> ()  [unwired: 2 in, 2 out]
          }
          frame True {
            n504 = property on="Auto Scroll" class="Bool (strict)"("BoolText.BGColor"=u32 16711680 ("Boolean Text.Text Colors:Text Color")) -> ()  [unwired: 2 in, 2 out]
          }
        }
      }
      event "Save Log": Value Change {
        n505 = event-data() -> ()  [unwired: 1 in, 6 out]
        n506 = call <vilib>:"Q.Enqueue Task.vi"("Task Name"="Save Log to File" ("Name"), "Q In"=w1226) -> ()  [unwired: 8 in, 2 out]
      }
    }
  }
